vi "Motors 1.vi"(2 "Motors Visa Ref":refnum<visa-resource-name>="COM7") -> ()   [LabVIEW 2010]
panel:
  out "output cluster":T1
  in  "Cluster":T2
  in  "Y Speed (mm/s)":dbl=1.0 min=0.0
  in  "Delta Y (mm)":dbl=1.0
  in  "Theta Speed (deg/s)":dbl=1.0 min=0.0
  in  "Delta Theta (deg)":dbl=1.0
  in  "(mm/s)":dbl min=0.4
  in  "(mm/s) 3":dbl min=0.4
  in  "(mm/s) 2":dbl min=4.0
  in  "(degrees/s)":dbl min=8.0
  in  "X Set Slew Speed":bool
  in  "Y Set Slew Speed":bool
  in  "Z Set Slew Speed":bool
  in  "Theta Set Slew Speed":bool
  in  "Go To Saved Position":bool
  in  "Defined Positions":i32(listbox)
  in  "Steps to deactivate hard limit after finding datums":dbl=500.0
  out "Loop i":i32
types:
  T1 = cluster{"Set Jogger?":refnum<vi>, "Normal":refnum<vi>, "Fast":refnum<vi>, "Jogger Axis":refnum<vi>, "X Multiplier":refnum<vi>, "Y Multiplier":refnum<vi>, "Z Multiplier":refnum<vi>, "Theta Multiplier":refnum<vi>, "Need to Update Motor Parameters":refnum<vi>}
  T2 = cluster{"Stop X?":refnum<vi>, "Stop Y?":refnum<vi>, "Stop Z?":refnum<vi>, "Stop Theta?":refnum<vi>, "Backlash?":refnum<vi>, "Backlash X":refnum<vi>, "Backlash Y":refnum<vi>, "Backlash Z":refnum<vi>, "Backlash Theta":refnum<vi>, "Manual IO?":refnum<vi>, "Manual Communication is Active\n(Close Before Ending Program)":refnum<vi>, "Reset Motors?":refnum<vi>, "Set Jogger?":refnum<vi>, "Normal":refnum<vi>, "Fast":refnum<vi>, "Jogger Axis":refnum<vi>, "Redefine Origin as Current Location?":refnum<vi>, "Save Current Motor Parameters?":refnum<vi>, "Find Datums Nearest Hard Limits?":refnum<vi>, "Saved Limits":refnum<vi>, "Use Datums Nearest Hard Limits to Reset Origin?":refnum<vi>, "X Go?":refnum<vi>, "Y Go?":refnum<vi>, "Z Go?":refnum<vi>, "Theta Go?":refnum<vi>, "Jog-Mode":refnum<vi>, "x+?":refnum<vi>, "x-?":refnum<vi>, "y+?":refnum<vi>, "y-?":refnum<vi>, "z+?":refnum<vi>, "z-?":refnum<vi>, "theta+?":refnum<vi>, "theta-?":refnum<vi>, "X Set Slew Speed?":refnum<vi>, "(mm/s)":refnum<vi>, "Y Set Slew Speed?":refnum<vi>, "(mm/s)":refnum<vi>, "Z Set Slew Speed?":refnum<vi>, "(mm/s)":refnum<vi>, "Theta Set Slew Speed?":refnum<vi>, "(degrees/s)":refnum<vi>, "Go To Saved Position?":refnum<vi>, "Defined Positions":refnum<vi>, "Need to Update Motor Parameters":refnum<vi>, "X Jogger Normal Speed":refnum<vi>, "X Jogger Fast Speed":refnum<vi>, "Y Jogger Normal Speed":refnum<vi>, "Y Jogger Fast Speed":refnum<vi>, "Z Jogger Normal Speed":refnum<vi>, "Z Jogger Fast Speed":refnum<vi>, "Theta Jogger Normal Speed":refnum<vi>, "Theta Jogger Fast Speed":refnum<vi>, "X Moving":refnum<vi>, "Y Moving":refnum<vi>, "Z Moving":refnum<vi>, "Theta Moving":refnum<vi>, "X Slew Speed (mm or degree/s)":refnum<vi>, "Y Slew Speed (mm or degree/s)":refnum<vi>, "Z Slew Speed (mm or degree/s)":refnum<vi>, "Theta Slew Speed (mm or degree/s)":refnum<vi>, "X-Axis (mm)":refnum<vi>, "Y-Axis (mm)":refnum<vi>, "Z-Axis (mm)":refnum<vi>, "Theta (deg)":refnum<vi>, "X Multiplier":refnum<vi>, "Y Multiplier":refnum<vi>, "Z Multiplier":refnum<vi>, "Theta Multiplier":refnum<vi>, "Motors Online":refnum<vi>, "Motors Status":refnum<vi>, "Status X":refnum<vi>, "Status Y":refnum<vi>, "Status Z":refnum<vi>, "Status Theta":refnum<vi>, "Motors error":refnum<vi>, "QUIT":refnum<vi>, "EMERGENCY":refnum<vi>, "X Go To":refnum<vi>, "Y Go To":refnum<vi>, "Z Go To":refnum<vi>, "Theta Go To":refnum<vi>, "Delta X (mm)":refnum<vi>, "Delta Y (mm)":refnum<vi>, "Delta Z (mm)":refnum<vi>, "Delta Theta (deg)":refnum<vi>, "X Speed (mm/s)":refnum<vi>, "Y Speed (mm/s)":refnum<vi>, "Z Speed (mm/s)":refnum<vi>, "Theta Speed (deg/s)":refnum<vi>, "x+":refnum<vi>, "x-":refnum<vi>, "y+":refnum<vi>, "y-":refnum<vi>, "z+":refnum<vi>, "z-":refnum<vi>, "theta+":refnum<vi>, "theta-":refnum<vi>}
  T3 = cluster{"Stop X?":refnum<vi>, "Stop Y?":refnum<vi>, "Stop Z?":refnum<vi>, "Stop Theta?":refnum<vi>}
  T4 = cluster{"Backlash?":refnum<vi>, "Backlash X":refnum<vi>, "Backlash Y":refnum<vi>, "Backlash Z":refnum<vi>, "Backlash Theta":refnum<vi>}
  T5 = cluster{"EMERGENCY":refnum<vi>, "Manual IO?":refnum<vi>, "Manual Communication is Active\n(Close Before Ending Program)":refnum<vi>, "Reset Motors?":refnum<vi>}
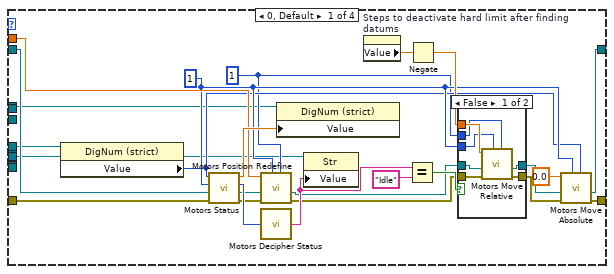
[diagram p4: hidden frame]
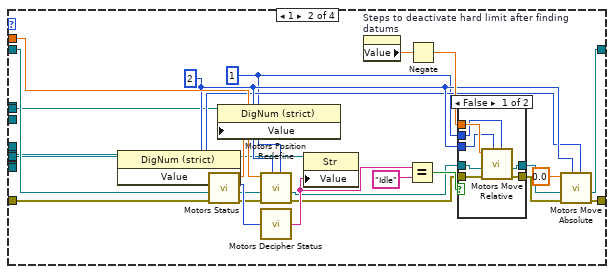
[diagram p6: hidden frame]
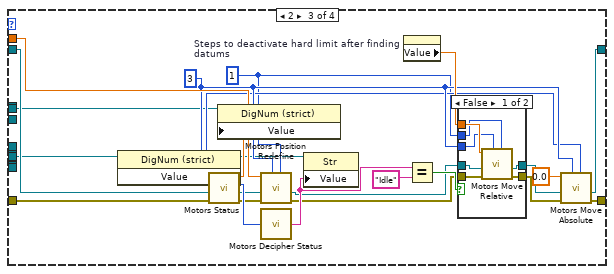
[diagram p8: hidden frame]
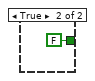
[diagram p12: hidden frame]
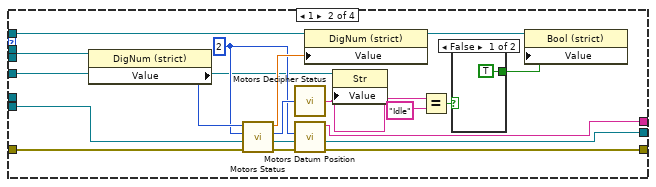
[diagram p13: hidden frame]
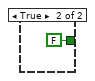
[diagram p14: hidden frame]
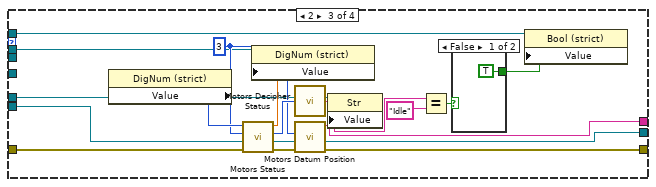
[diagram p15: hidden frame]
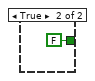
[diagram p16: hidden frame]
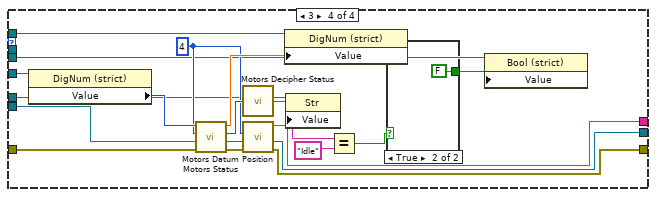
[diagram p17: hidden frame]
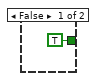
[diagram p18: hidden frame]
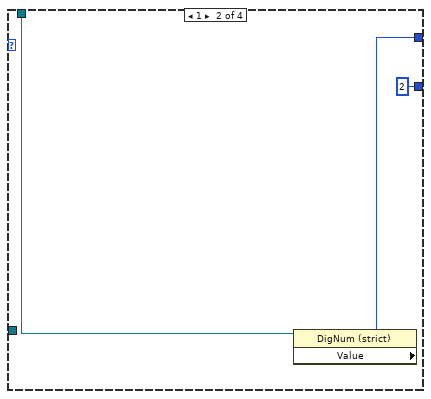
[diagram p19: hidden frame]
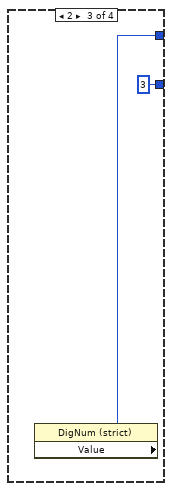
[diagram p20: hidden frame]
diagram:
  n1 = Unbundle("Cluster") -> ("Stop X?"=w27:refnum<vi>, "Stop Y?"=w26:refnum<vi>, "Stop Z?"=w25:refnum<vi>, "Stop Theta?"=w24:refnum<vi>, "Backlash?"=w23:refnum<vi>, "Backlash X"=w22:refnum<vi>, "Backlash Y"=w21:refnum<vi>, "Backlash Z"=w20:refnum<vi>, "Backlash Theta"=w19:refnum<vi>, "Manual IO?"=w17:refnum<vi>, "Manual Communication is Active\n(Close Before Ending Program)"=w16:refnum<vi>, "Reset Motors?"=w15:refnum<vi>, "Set Jogger?"=w10:refnum<vi>, "Normal"=w9:refnum<vi>, "Fast"=w8:refnum<vi>, "Jogger Axis"=w7:refnum<vi>, "Redefine Origin as Current Location?"=w68:refnum<vi>, "Save Current Motor Parameters?"=w67:refnum<vi>, "Find Datums Nearest Hard Limits?"=w66:refnum<vi>, "Saved Limits"=w65:refnum<vi>, "Use Datums Nearest Hard Limits to Reset Origin?"=w64:refnum<vi>, "X Go?"=w55:refnum<vi>, "Y Go?"=w52:refnum<vi>, "Z Go?"=w51:refnum<vi>, "Theta Go?"=w49:refnum<vi>, "Jog-Mode"=w47:refnum<vi>, "x+?"=w40:refnum<vi>, "x-?"=w41:refnum<vi>, "y+?"=w39:refnum<vi>, "y-?"=w38:refnum<vi>, "Need to Update Motor Parameters"=w1:refnum<vi>, "X Moving"=w46:refnum<vi>, "Y Moving"=w29:refnum<vi>, "Z Moving"=w63:refnum<vi>, "Theta Moving"=w62:refnum<vi>, "X-Axis (mm)"=w43:refnum<vi>, "Y-Axis (mm)"=w36:refnum<vi>, "Z-Axis (mm)"=w61:refnum<vi>, "Theta (deg)"=w59:refnum<vi>, "X Multiplier"=w6:refnum<vi>, "Y Multiplier"=w5:refnum<vi>, "Z Multiplier"=w4:refnum<vi>, "Theta Multiplier"=w2:refnum<vi>, "Motors Online"=w69:refnum<vi>, "Motors Status"=w71:refnum<vi>, "Status X"=w42:refnum<vi>, "Status Y"=w30:refnum<vi>, "Status Z"=w60:refnum<vi>, "Status Theta"=w58:refnum<vi>, "Motors error"=w13:refnum<vi>, "QUIT"=w73:refnum<vi>, "EMERGENCY"=w14:refnum<vi>, "X Go To"=w54:refnum<vi>, "Y Go To"=w53:refnum<vi>, "Z Go To"=w50:refnum<vi>, "Theta Go To"=w48:refnum<vi>, "Delta X (mm)"=w45:refnum<vi>, "Delta Y (mm)"=w28:refnum<vi>, "X Speed (mm/s)"=w44:refnum<vi>, "Y Speed (mm/s)"=w37:refnum<vi>, "x+"=w34:refnum<vi>, "x-"=w33:refnum<vi>, "y+"=w32:refnum<vi>, "y-"=w31:refnum<vi>)  [unwired: 34 out]
  n2 = property on="Property Node" class="Bool (strict)"(reference=w1, "Value"=TRUE) -> (reference out=w57:refnum<vi>)  [unwired: 1 in, 1 out]
  n3 = Bundle("Stop X?"=w27, "Stop Y?"=w26, "Stop Z?"=w25, "Stop Theta?"=w24) -> (w12:T3)  [unwired: 1 in]
  n4 = Bundle("Backlash?"=w23, "Backlash X"=w22, "Backlash Y"=w21, "Backlash Z"=w20, "Backlash Theta"=w19) -> (w18:T4)  [unwired: 1 in]
  n5 = Bundle("EMERGENCY"=w14, "Manual IO?"=w17, "Manual Communication is Active\n(Close Before Ending Program)"=w16, "Reset Motors?"=w15) -> (w11:T5)  [unwired: 1 in]
  n6 = Bundle("Set Jogger?"=w10, "Normal"=w9, "Fast"=w8, "Jogger Axis"=w7, "X Multiplier"=w6, "Y Multiplier"=w5, "Z Multiplier"=w4, "Theta Multiplier"=w2, "Need to Update Motor Parameters"=w1) -> (w3:T1)  [unwired: 1 in]
  "output cluster" <- w3
  n7 = call "Motors Open.vi"("VISA in"="Motors Visa Ref") -> ("error out"=w77:errorcluster, "VISA out"=w74:refnum<visa-resource-name>)  [unwired: 1 in]
  n8 = call <vilib>:"Simple Error Handler.vi"("error in (no error)"=w77) -> ("error?"=w76:bool, "error out"=w78:errorcluster)  [unwired: 4 in, 3 out]
  n9 = property on="Property Node" class="Str"(reference=w71, "Value"="Opening Communications") -> (reference out=w72:refnum<vi>)  [unwired: 1 in, 1 out]
  n10 = property on="Property Node" class="Clust (strict)"(reference=w13, "Value"=w78) -> ()  [unwired: 1 in, 2 out]
  n11 = Not(x=w76) -> (.not. x?=w75:bool)
  n12 = case shown="True" w75 {
    tunnel: w72 -> [_ w153]
    tunnel: w74 -> [_ w152]
    tunnel: w13 -> [_ w151]
    tunnel: w73 -> [_ w150]
    tunnel: w14 -> [_ w149]
    tunnel: w6 -> [_ w148]
    tunnel: w5 -> [_ w147]
    tunnel: w2 -> [_ w146]
    tunnel: w57 -> [_ w145]
    tunnel: w68 -> [_ w144]
    tunnel: w67 -> [_ w143]
    tunnel: w66 -> [_ w142]
    tunnel: w6 -> [_ w140]
    tunnel: w43 -> [_ w139]
    tunnel: w42 -> [_ w138]
    tunnel: w46 -> [_ w137]
    tunnel: w65 -> [_ w136]
    tunnel: w64 -> [_ w135]
    tunnel: w29 -> [_ w134]
    tunnel: w63 -> [_ w133]
    tunnel: w62 -> [_ w132]
    tunnel: w6 -> [_ w131]
    tunnel: w5 -> [_ w130]
    tunnel: w2 -> [_ w129]
    tunnel: w43 -> [_ w128]
    tunnel: w36 -> [_ w127]
    tunnel: w61 -> [_ w126]
    tunnel: w42 -> [_ w125]
    tunnel: w30 -> [_ w124]
    tunnel: w60 -> [_ w123]
    tunnel: w59 -> [_ w122]
    tunnel: w58 -> [_ w121]
    tunnel: w55 -> [_ w120]
    tunnel: w6 -> [_ w119]
    tunnel: w54 -> [_ w118]
    tunnel: w5 -> [_ w117]
    tunnel: w53 -> [_ w116]
    tunnel: w52 -> [_ w115]
    tunnel: w51 -> [_ w114]
    tunnel: w50 -> [_ w113]
    tunnel: w49 -> [_ w112]
    tunnel: w2 -> [_ w111]
    tunnel: w48 -> [_ w110]
    tunnel: w41 -> [_ w109]
    tunnel: w47 -> [_ w108]
    tunnel: w46 -> [_ w107]
    tunnel: w45 -> [_ w106]
    tunnel: w6 -> [_ w105]
    tunnel: w44 -> [_ w104]
    tunnel: w43 -> [_ w103]
    tunnel: w40 -> [_ w102]
    tunnel: w41 -> [_ w101]
    tunnel: w42 -> [_ w100]
    tunnel: w41 -> [_ w99]
    tunnel: w40 -> [_ w98]
    tunnel: w40 -> [_ w97]
    tunnel: w39 -> [_ w96]
    tunnel: w38 -> [_ w95]
    tunnel: w5 -> [_ w94]
    tunnel: w37 -> [_ w93]
    tunnel: w36 -> [_ w92]
    tunnel: w34 -> [_ w91]
    tunnel: w33 -> [_ w90]
    tunnel: w32 -> [_ w89]
    tunnel: w31 -> [_ w88]
    tunnel: w30 -> [_ w87]
    tunnel: w29 -> [_ w86]
    tunnel: w28 -> [_ w85]
    tunnel: w5 -> [_ w84]
    tunnel: w18 -> [_ w83]
    tunnel: w12 -> [_ w82]
    tunnel: w11 -> [_ w81]
    tunnel: w3 -> [_ w80]
    frame False {
    }
    frame True {
      n13 = property on="Property Node" class="Str"(reference=w153, "Value"="Running") -> (reference out=w141:refnum<vi>)  [unwired: 1 in, 1 out]
      n14 = while {
        shift-right: _ -> [_]
        shift-left: w152 -> [w166]
        tunnel: w151 -> [w321]
        tunnel: w150 -> [w259]
        tunnel: w149 -> [_]
        tunnel: w148 -> [w256]
        tunnel: w147 -> [w255]
        tunnel: w146 -> [w254]
        tunnel: w145 -> [w253]
        tunnel: w144 -> [w251]
        tunnel: w143 -> [w250]
        tunnel: w142 -> [w248]
        tunnel: w141 -> [w247]
        tunnel: w140 -> [w246]
        tunnel: w139 -> [w245]
        tunnel: w138 -> [w244]
        tunnel: w137 -> [w243]
        tunnel: w136 -> [w242]
        tunnel: w135 -> [w222]
        tunnel: w134 -> [w240]
        tunnel: w133 -> [w239]
        tunnel: w132 -> [w238]
        tunnel: w131 -> [w235]
        tunnel: w130 -> [w234]
        tunnel: w129 -> [w233]
        tunnel: w128 -> [w232]
        tunnel: w127 -> [w231]
        tunnel: w126 -> [w230]
        tunnel: w125 -> [w229]
        tunnel: w124 -> [w228]
        tunnel: w123 -> [w227]
        tunnel: w122 -> [w226]
        tunnel: w121 -> [w225]
        tunnel: w120 -> [w223]
        tunnel: w119 -> [w214]
        tunnel: w118 -> [w213]
        tunnel: w117 -> [w212]
        tunnel: w116 -> [w211]
        tunnel: w115 -> [w209]
        tunnel: w114 -> [w206]
        tunnel: w113 -> [w204]
        tunnel: w112 -> [w202]
        tunnel: w111 -> [w198]
        tunnel: w110 -> [w200]
        tunnel: w109 -> [w199]
        tunnel: w108 -> [w196]
        tunnel: w107 -> [w195]
        tunnel: w106 -> [w194]
        tunnel: w105 -> [w193]
        tunnel: w104 -> [w192]
        tunnel: w103 -> [w191]
        tunnel: w102 -> [w190]
        tunnel: w101 -> [w189]
        tunnel: w100 -> [w188]
        tunnel: w99 -> [w187]
        tunnel: w98 -> [w186]
        tunnel: w97 -> [w185]
        tunnel: w96 -> [w184]
        tunnel: w95 -> [w183]
        tunnel: w94 -> [w182]
        tunnel: w93 -> [w181]
        tunnel: w92 -> [w180]
        tunnel: w91 -> [w176]
        tunnel: w90 -> [w175]
        tunnel: w89 -> [w174]
        tunnel: w88 -> [w173]
        tunnel: w87 -> [w172]
        tunnel: w86 -> [w169]
        tunnel: w85 -> [w168]
        tunnel: w84 -> [w167]
        tunnel: w83 -> [w162]
        tunnel: w82 -> [w164]
        tunnel: w81 -> [w160]
        tunnel: w80 -> [w155]
        i -> [w260]
        stop <- w322 stop-if-true
        # "This loop contains all of the code that has to communicate directly with the manipulator motor controllers.  They are arranged linearly to ensure multiple serial I/O's are never attempted simultaneously.  Note that this loop executes very slowly (each serial I/O takes about 1/20 sec)."
        n15 = property on="Property Node" class="Bool (strict)"(reference=w184) -> (reference out=w170:refnum<vi>, "Value"=w272:bool)  [unwired: 1 in, 1 out]
        n16 = property on="Property Node" class="Bool (strict)"(reference=w183) -> (reference out=w171:refnum<vi>, "Value"=w273:bool)  [unwired: 1 in, 1 out]
        n17 = property on="Property Node" class="Clust (strict)"(reference=w321) -> ("Value"=w163:errorcluster)  [unwired: 1 in, 2 out]
        n18 = Or(x=w272, y=w273) -> (x .or. y?=w303:bool)
        n19 = property on="Property Node" class="Bool (strict)"(reference=w199) -> (reference out=w178:refnum<vi>, "Value"=w276:bool)  [unwired: 1 in, 1 out]
        n20 = property on="Property Node" class="Bool (strict)"(reference=w186) -> (reference out=w177:refnum<vi>, "Value"=w277:bool)  [unwired: 1 in, 1 out]
        n21 = call "Motors Sub 01.vi"("Cluster"=w164, "Error In"=w163, "VISA in"=w166) -> ("error out"=w161:errorcluster, "VISA out"=w165:refnum<visa-resource-name>)  [unwired: 7 in]
        n22 = property on="Property Node" class="Bool (strict)"(reference=w196) -> ("Value"=w197:bool)  [unwired: 1 in, 2 out]
        n23 = call "Motors Sub 02.vi"("Cluster"=w162, "error in"=w161, "VISA in"=w165) -> ("error out"=w158:errorcluster, "VISA out"=w159:refnum<visa-resource-name>)  [unwired: 7 in]
        n24 = property on="Property Node" class="Bool (strict)"(reference=w223) -> (reference out=w179:refnum<vi>, "Value"=w224:bool)  [unwired: 1 in, 1 out]
        n25 = property on="Property Node" class="Bool (strict)"(reference=w259) -> ("Value"=w322:bool)  [unwired: 1 in, 2 out]
        n26 = Or(x=w277, y=w276) -> (x .or. y?=w309:bool)
        n27 = call "Motors Sub 03.vi"("Cluster"=w160, "error in"=w158, "VISA in"=w159) -> ("error out"=w156:errorcluster, "VISA out"=w157:refnum<visa-resource-name>)  [unwired: 7 in]
        n28 = property on="Property Node" class="DigNum (strict)" props=["Value"]() -> ()  [unwired: 2 in, 3 out]
        n29 = call "Motors Sub 04.vi"("Cluster"=w155, "error in"=w156, "VISA in"=w157) -> ()  [unwired: 7 in, 2 out]
        n30 = property on="Property Node" class="Bool (strict)"(reference=w209) -> (reference out=w208:refnum<vi>, "Value"=w210:bool)  [unwired: 1 in, 1 out]
        n31 = property on="Property Node" class="Bool (strict)"(reference=w206) -> (reference out=w205:refnum<vi>, "Value"=w207:bool)  [unwired: 1 in, 1 out]
        n32 = property on="Property Node" class="Bool (strict)"(reference=w202) -> (reference out=w201:refnum<vi>, "Value"=w203:bool)  [unwired: 1 in, 1 out]
        n33 = property on="Property Node" class="Ring (strict)"() -> ("Value"=w257:u16)  [unwired: 2 in, 2 out]
        n34 = property on="Property Node" class="Bool (strict)"() -> ("Value"=w274:bool)  [unwired: 2 in, 2 out]
        n35 = property on="Property Node" class="Bool (strict)"() -> ("Value"=w275:bool)  [unwired: 2 in, 2 out]
        n36 = case shown="0, Default" w257 {
          tunnel: [u32 1 u32 2 u32 3 u32 4] -> w269
          tunnel: [w719 w722 w724 w727] -> w268
          tunnel: w256 -> [w718 _ _ _]
          tunnel: w255 -> [_ w721 _ _]
          tunnel: w254 -> [_ _ _ w726]
          frame 0, Default {
            n37 = property on="Property Node" class="DigNum (strict)"(reference=w718) -> ("Value"=w719:u32)  [unwired: 1 in, 2 out]
          }
          frame 1 {
            n38 = property on="Property Node" class="DigNum (strict)"(reference=w721) -> ("Value"=w722:u32)  [unwired: 1 in, 2 out]
          }
          frame 2 {
            n39 = property on="Property Node" class="DigNum (strict)"() -> ("Value"=w724:u32)  [unwired: 2 in, 2 out]
          }
          frame 3 {
            n40 = property on="Property Node" class="DigNum (strict)"(reference=w726) -> ("Value"=w727:u32)  [unwired: 1 in, 2 out]
          }
        }
        n41 = Or(x=w275, y=w274) -> (x .or. y?=w306:bool)
        n42 = property on="Property Node" class="Bool (strict)"() -> (reference out=w215:refnum<vi>, "Value"=w258:bool)  [unwired: 2 in, 1 out]
        n43 = case shown="True" w258 {
          tunnel: [_ w1371] -> w319
          tunnel: [_ w1368] -> w320
          tunnel: w269 -> [_ w1370]
          tunnel: w268 -> [_ w1369]
          tunnel: w253 -> [_ w1366]
          tunnel: w215 -> [_ w1362]
          frame False {
          }
          frame True {
            n44 = property on="Property Node" class="DigNum (strict)"() -> ("Value"=w1365:dbl)  [unwired: 2 in, 2 out]
            n45 = property on="Property Node" class="DigNum (strict)"() -> ("Value"=w1364:dbl)  [unwired: 2 in, 2 out]
            n46 = property on="Property Node" class="Bool (strict)"(reference=w1366, "Value"=TRUE ("Need to Update Motor Parameters")) -> ()  [unwired: 1 in, 2 out]
            n47 = call "Motors Jogger Speed.vi"("Axis Multiplier"=w1369, "Axis"=w1370, "Fast Speed (mm or degree/sec)"=w1364, "Normal Speed (mm or degree/sec)"=w1365) -> ("error out"=w1371:errorcluster, "VISA out"=w1368:refnum<visa-resource-name>)  [unwired: 6 in]
            n48 = property on="Property Node" class="Bool (strict)"(reference=w1362, "Value"=FALSE) -> ()  [unwired: 1 in, 2 out]
          }
        }
        n49 = property on="Property Node" class="Bool (strict)"(reference=w251) -> (reference out=w216:refnum<vi>, "Value"=w252:bool)  [unwired: 1 in, 1 out]
        n50 = property on="Property Node" class="Bool (strict)"(reference=w250) -> (reference out=w218:refnum<vi>, "Value"=w217:bool)  [unwired: 1 in, 1 out]
        n51 = case shown="True" w252 {
          tunnel: w320 -> [w1354 w1361]
          tunnel: w319 -> [w1355 w1357]
          tunnel: [w1355 w1359] -> w219
          tunnel: [w1354 w1360] -> w318
          tunnel: w216 -> [_ w1356]
          frame False {
          }
          frame True {
            n52 = property on="Property Node" class="Bool (strict)"(reference=w1356, "Value"=FALSE) -> ()  [unwired: 1 in, 2 out]
            n53 = call "Motors Redefine Origin.vi"("error in"=w1357, "VISA in"=w1361) -> ("error out"=w1359:errorcluster, "VISA out"=w1360:refnum<visa-resource-name>)
          }
        }
        n54 = property on="Property Node" class="Bool (strict)"(reference=w248) -> (reference out=w221:refnum<vi>, "Value"=w249:bool)  [unwired: 1 in, 1 out]
        n55 = case shown="True" w217 {
          tunnel: w219 -> [w1347 w1353]
          tunnel: [w1347 w1352] -> w266
          tunnel: w318 -> [w1346 w1351]
          tunnel: [w1346 w1350] -> w265
          tunnel: w218 -> [_ w1349]
          frame False {
          }
          frame True {
            n56 = property on="Property Node" class="Bool (strict)"(reference=w1349, "Value"=FALSE) -> ()  [unwired: 1 in, 2 out]
            n57 = call "Motors Save.vi"("error in"=w1353, "VISA in"=w1351) -> ("error out"=w1352:errorcluster, "VISA out"=w1350:refnum<visa-resource-name>)
          }
        }
        n58 = case shown="True" w249 {
          tunnel: w266 -> [w536 w566]
          tunnel: [w536 w564] -> w263
          tunnel: [w535 w565] -> w261
          tunnel: w265 -> [w535 w567]
          tunnel: w247 -> [w533 w559]
          tunnel: w246 -> [_ w556]
          tunnel: w245 -> [_ w555]
          tunnel: w244 -> [_ w554]
          tunnel: w243 -> [_ w553]
          tunnel: w242 -> [w534 w552]
          tunnel: w234 -> [_ w551]
          tunnel: w231 -> [_ w550]
          tunnel: w228 -> [_ w549]
          tunnel: w240 -> [_ w548]
          tunnel: w230 -> [_ w547]
          tunnel: w227 -> [_ w546]
          tunnel: w239 -> [_ w545]
          tunnel: w233 -> [_ w544]
          tunnel: w226 -> [_ w543]
          tunnel: w225 -> [_ w542]
          tunnel: w238 -> [_ w541]
          tunnel: [w534 w540] -> w237
          tunnel: [w533 w539] -> w236
          tunnel: w221 -> [_ w538]
          frame False {
          }
          frame True {
            n59 = flat-sequence {
              tunnel: w566 -> [w572]
              tunnel: w567 -> [w573]
              tunnel: [w573] -> w563
              tunnel: [w572] -> w562
              tunnel: w559 -> [w569]
              tunnel: [w568] -> w557
              tunnel: w563 -> [w608]
              tunnel: w562 -> [w607]
              tunnel: [w603] -> w561
              tunnel: [w602] -> w560
              tunnel: [w592] -> w558
              tunnel: w557 -> [w592]
              tunnel: w556 -> [w591]
              tunnel: w555 -> [w590]
              tunnel: w554 -> [w589]
              tunnel: w553 -> [w588]
              tunnel: w552 -> [w586]
              tunnel: w551 -> [w585]
              tunnel: w550 -> [w584]
              tunnel: w549 -> [w583]
              tunnel: w548 -> [w582]
              tunnel: w547 -> [w581]
              tunnel: w546 -> [w580]
              tunnel: w545 -> [w579]
              tunnel: w544 -> [w578]
              tunnel: w543 -> [w577]
              tunnel: w542 -> [w576]
              tunnel: w541 -> [w575]
              tunnel: [w574] -> w540
              tunnel: [w716] -> w564
              tunnel: [w717] -> w565
              tunnel: w561 -> [w717]
              tunnel: w560 -> [w716]
              tunnel: w558 -> [w714]
              tunnel: [w713] -> w539
              frame #0 {
                n60 = call <vilib>:"Set Busy.vi"("disable click? (T)"=FALSE) -> ()  [unwired: 9 in, 2 out]
                n61 = property on="Property Node" class="Str"(reference=w569, "Value"="Finding Datums Nearest Hard Limits\nThis May Take a Few Minutes" ("Status")) -> (reference out=w568:refnum<vi>)  [unwired: 1 in, 1 out]
              }
              frame #1 {
                n62 = call "Motors Find Datums.vi"("error in"=w607, "VISA in"=w608) -> ("error out"=w604:errorcluster, "VISA out"=w605:refnum<visa-resource-name>)
                n63 = for {
                  N: 4 -> [_]
                  shift-right: [w627] -> w602
                  shift-left: w604 -> [w628]
                  shift-right: [w626] -> w603
                  shift-left: w605 -> [w629]
                  tunnel: [w625] -> w594 mode=indexing
                  tunnel: w591 -> [w623]
                  tunnel: w590 -> [w622]
                  tunnel: w589 -> [w621]
                  tunnel: w588 -> [w620]
                  tunnel: w585 -> [w619]
                  tunnel: w584 -> [w618]
                  tunnel: w583 -> [w617]
                  tunnel: w582 -> [w616]
                  tunnel: w581 -> [w615]
                  tunnel: w580 -> [w614]
                  tunnel: w579 -> [w613]
                  tunnel: w578 -> [w612]
                  tunnel: w577 -> [w611]
                  tunnel: w576 -> [w610]
                  tunnel: w575 -> [w609]
                  i -> [w624]
                  n64 = case shown="0, Default" w624 {
                    tunnel: w628 -> [w642 w663 w683 w704]
                    tunnel: w629 -> [w643 w664 w684 w705]
                    tunnel: [w636 w657 w676 w697] -> w627
                    tunnel: [w637 w658 w677 w698] -> w626
                    tunnel: [w634 w655 w680 w701] -> w625
                    tunnel: w623 -> [w633 _ _ _]
                    tunnel: w622 -> [w632 _ _ _]
                    tunnel: w621 -> [w631 _ _ _]
                    tunnel: w620 -> [w630 _ _ _]
                    tunnel: w619 -> [_ w654 _ _]
                    tunnel: w618 -> [_ w653 _ _]
                    tunnel: w617 -> [_ w652 _ _]
                    tunnel: w616 -> [_ w651 _ _]
                    tunnel: w615 -> [_ _ w674 _]
                    tunnel: w614 -> [_ _ w673 _]
                    tunnel: w613 -> [_ _ w672 _]
                    tunnel: w612 -> [_ _ _ w695]
                    tunnel: w611 -> [_ _ _ w694]
                    tunnel: w610 -> [_ _ _ w693]
                    tunnel: w609 -> [_ _ _ w692]
                    frame 0, Default {
                      w635 = 1 ("Axis")
                      n65 = property on="Property Node" class="DigNum (strict)"(reference=w633) -> ("Value"=w641:u32)  [unwired: 1 in, 2 out]
                      n66 = call "Motors Status.vi"("error in"=w642, "VISA in"=w643, "Axis"=w635, "Axis Multiplier"=w641) -> ("error out"=w638:errorcluster, "VISA out"=w639:refnum<visa-resource-name>, "OS"=w648:i32, "Actual Position (mm or deg)"=w640:dbl)  [unwired: 3 in]
                      n67 = property on="Property Node" class="DigNum (strict)"(reference=w632, "Value"=w640) -> ()  [unwired: 1 in, 2 out]
                      n68 = call "Motors Decipher Status.vi"("OS"=w648) -> ("Status"=w647:string)
                      n69 = call "Motors Datum Position.vi"("error in"=w638, "VISA in"=w639, "Axis"=w635) -> ("error out"=w636:errorcluster, "VISA out"=w637:refnum<visa-resource-name>, "Datum Position (steps)"=w634:string)  [unwired: 5 in]
                      n70 = property on="Property Node" class="Str"(reference=w631, "Value"=w647) -> ()  [unwired: 1 in, 2 out]
                      n71 = Equal?(x=w647, y="Idle") -> (x = y?=w645:bool)
                      n72 = case shown="False" w645 {
                        tunnel: [TRUE FALSE] -> w644
                        frame False {
                        }
                        frame True {
                        }
                      }
                      n73 = property on="Property Node" class="Bool (strict)"(reference=w630, "Value"=w644) -> ()  [unwired: 1 in, 2 out]
                    }
                    frame 1 {
                      w656 = 2 ("Axis")
                      n74 = property on="Property Node" class="DigNum (strict)"(reference=w654) -> ("Value"=w662:u32)  [unwired: 1 in, 2 out]
                      n75 = call "Motors Status.vi"("error in"=w663, "VISA in"=w664, "Axis"=w656, "Axis Multiplier"=w662) -> ("error out"=w659:errorcluster, "VISA out"=w660:refnum<visa-resource-name>, "OS"=w669:i32, "Actual Position (mm or deg)"=w661:dbl)  [unwired: 3 in]
                      n76 = call "Motors Decipher Status.vi"("OS"=w669) -> ("Status"=w667:string)
                      n77 = call "Motors Datum Position.vi"("error in"=w659, "VISA in"=w660, "Axis"=w656) -> ("error out"=w657:errorcluster, "VISA out"=w658:refnum<visa-resource-name>, "Datum Position (steps)"=w655:string)  [unwired: 5 in]
                      n78 = property on="Property Node" class="DigNum (strict)"(reference=w653, "Value"=w661) -> ()  [unwired: 1 in, 2 out]
                      n79 = property on="Property Node" class="Str"(reference=w652, "Value"=w667) -> ()  [unwired: 1 in, 2 out]
                      n80 = Equal?(x=w667, y="Idle") -> (x = y?=w666:bool)
                      n81 = case shown="False" w666 {
                        tunnel: [TRUE FALSE] -> w665
                        frame False {
                        }
                        frame True {
                        }
                      }
                      n82 = property on="Property Node" class="Bool (strict)"(reference=w651, "Value"=w665) -> ()  [unwired: 1 in, 2 out]
                    }
                    frame 2 {
                      w675 = 3 ("Axis")
                      n83 = property on="Property Node" class="DigNum (strict)"() -> ("Value"=w682:u32)  [unwired: 2 in, 2 out]
                      n84 = call "Motors Status.vi"("error in"=w683, "VISA in"=w684, "Axis"=w675, "Axis Multiplier"=w682) -> ("error out"=w678:errorcluster, "VISA out"=w679:refnum<visa-resource-name>, "OS"=w689:i32, "Actual Position (mm or deg)"=w681:dbl)  [unwired: 3 in]
                      n85 = property on="Property Node" class="DigNum (strict)"(reference=w674, "Value"=w681) -> ()  [unwired: 1 in, 2 out]
                      n86 = call "Motors Decipher Status.vi"("OS"=w689) -> ("Status"=w687:string)
                      n87 = call "Motors Datum Position.vi"("error in"=w678, "VISA in"=w679, "Axis"=w675) -> ("error out"=w676:errorcluster, "VISA out"=w677:refnum<visa-resource-name>, "Datum Position (steps)"=w680:string)  [unwired: 5 in]
                      n88 = property on="Property Node" class="Str"(reference=w673, "Value"=w687) -> ()  [unwired: 1 in, 2 out]
                      n89 = Equal?(x=w687, y="Idle") -> (x = y?=w686:bool)
                      n90 = case shown="False" w686 {
                        tunnel: [TRUE FALSE] -> w685
                        frame False {
                        }
                        frame True {
                        }
                      }
                      n91 = property on="Property Node" class="Bool (strict)"(reference=w672, "Value"=w685) -> ()  [unwired: 1 in, 2 out]
                    }
                    frame 3 {
                      w696 = 4 ("Axis")
                      n92 = property on="Property Node" class="DigNum (strict)"(reference=w695) -> ("Value"=w703:u32)  [unwired: 1 in, 2 out]
                      n93 = call "Motors Status.vi"("error in"=w704, "VISA in"=w705, "Axis"=w696, "Axis Multiplier"=w703) -> ("error out"=w699:errorcluster, "VISA out"=w700:refnum<visa-resource-name>, "OS"=w710:i32, "Actual Position (mm or deg)"=w702:dbl)  [unwired: 3 in]
                      n94 = call "Motors Decipher Status.vi"("OS"=w710) -> ("Status"=w708:string)
                      n95 = call "Motors Datum Position.vi"("error in"=w699, "VISA in"=w700, "Axis"=w696) -> ("error out"=w697:errorcluster, "VISA out"=w698:refnum<visa-resource-name>, "Datum Position (steps)"=w701:string)  [unwired: 5 in]
                      n96 = property on="Property Node" class="DigNum (strict)"(reference=w694, "Value"=w702) -> ()  [unwired: 1 in, 2 out]
                      n97 = property on="Property Node" class="Str"(reference=w693, "Value"=w708) -> ()  [unwired: 1 in, 2 out]
                      n98 = Equal?(x=w708, y="Idle") -> (x = y?=w707:bool)
                      n99 = case shown="True" w707 {
                        tunnel: [TRUE FALSE] -> w706
                        frame False {
                        }
                        frame True {
                        }
                      }
                      n100 = property on="Property Node" class="Bool (strict)"(reference=w692, "Value"=w706) -> ()  [unwired: 1 in, 2 out]
                    }
                  }
                }
                n101 = Build Array (concatenate)("Limits", w594) -> (w593:string[])
                n102 = Initialize Array("", 0 ("dimension size"), 0 ("dimension size")) -> (w600:string[][])
                n103 = Build Array (concatenate)(w593, w600) -> (w598:string[][])
                n104 = property on="Property Node" class="Path"(reference=w586) -> (reference out=w574:refnum<vi>, "Value"=w587:path)  [unwired: 1 in, 1 out]
                n105 = Transpose 2D Array(2D array=w598) -> (transposed array=w597:string[][])
                n106 = call "Motors Position Rewrite.vi"("file path"=w587, "Array of Positions"=w597) -> ()  [unwired: 9 in]
              }
              frame #2 {
                n107 = call <vilib>:"Unset Busy.vi"() -> ()  [unwired: 11 in, 1 out]
                n108 = property on="Property Node" class="Str"(reference=w714, "Value"="Running" ("Status")) -> (reference out=w713:refnum<vi>)  [unwired: 1 in, 1 out]
              }
            }
            n109 = property on="Property Node" class="Bool (strict)"(reference=w538, "Value"=FALSE) -> ()  [unwired: 1 in, 2 out]
          }
        }
        n110 = property on="Property Node" class="Bool (strict)"(reference=w222) -> (reference out=w220:refnum<vi>, "Value"=w241:bool)  [unwired: 1 in, 1 out]
        n111 = case shown="True" w241 {
          tunnel: [w325 w345] -> w264
          tunnel: w263 -> [w325 w347]
          tunnel: [w324 w344] -> w262
          tunnel: w261 -> [w324 w348]
          tunnel: w237 -> [_ w343]
          tunnel: w236 -> [w323 w328]
          tunnel: w235 -> [_ w342]
          tunnel: w234 -> [_ w341]
          tunnel: w233 -> [_ w340]
          tunnel: w232 -> [_ w339]
          tunnel: w231 -> [_ w338]
          tunnel: w230 -> [_ w337]
          tunnel: w229 -> [_ w336]
          tunnel: w228 -> [_ w335]
          tunnel: w227 -> [_ w334]
          tunnel: w226 -> [_ w333]
          tunnel: w225 -> [_ w332]
          tunnel: [w323 w329] -> _
          tunnel: w220 -> [_ w327]
          frame False {
          }
          frame True {
            n112 = property on="Property Node" class="Bool (strict)"(reference=w327, "Value"=FALSE) -> ()  [unwired: 1 in, 2 out]
            n113 = flat-sequence {
              tunnel: w347 -> [w352]
              tunnel: [w352] -> w346
              tunnel: w328 -> [w350]
              tunnel: [w349] -> w330
              tunnel: w348 -> [w375]
              tunnel: w346 -> [w376]
              tunnel: [w371] -> w345
              tunnel: [w370] -> w344
              tunnel: w343 -> [w366]
              tunnel: w342 -> [w364]
              tunnel: w341 -> [w363]
              tunnel: w340 -> [w362]
              tunnel: w339 -> [w361]
              tunnel: w338 -> [w360]
              tunnel: w337 -> [w359]
              tunnel: w336 -> [w358]
              tunnel: w335 -> [w357]
              tunnel: w334 -> [w356]
              tunnel: w333 -> [w355]
              tunnel: w332 -> [w354]
              tunnel: [w353] -> w331
              tunnel: w330 -> [w353]
              tunnel: w331 -> [w531]
              tunnel: [w530] -> w329
              frame #0 {
                n114 = call <vilib>:"Set Busy.vi"() -> ()  [unwired: 10 in, 2 out]
                n115 = property on="Property Node" class="Str"(reference=w350, "Value"="Finding Datums Nearest Hard Limits\nThis May Take a Few Minutes" ("Status")) -> (reference out=w349:refnum<vi>)  [unwired: 1 in, 1 out]
              }
              frame #1 {
                n116 = property on="Property Node" class="Path"(reference=w366) -> ("Value"=w365:path)  [unwired: 1 in, 2 out]
                n117 = call "Motors Find Datums.vi"("error in"=w376, "VISA in"=w375) -> ("error out"=w373:errorcluster, "VISA out"=w374:refnum<visa-resource-name>)
                n118 = call "Motors Position Load.vi"("error in"=w373, "file path"=w365) -> ("error out"=w372:errorcluster, "Positions"=w369:string[][])
                n119 = Delete From Array(array=w369, index (row)=0) -> (array with subset deleted=w367:string[][])  [unwired: 2 in, 1 out]
                n120 = for {
                  shift-right: [w394] -> w371
                  shift-left: w372 -> [w395]
                  shift-right: [w393] -> w370
                  shift-left: w374 -> [w396]
                  tunnel: w367 -> [w392] mode=indexing
                  tunnel: w364 -> [w387]
                  tunnel: w363 -> [w386]
                  tunnel: w362 -> [w385]
                  tunnel: w361 -> [w384]
                  tunnel: w360 -> [w383]
                  tunnel: w359 -> [w382]
                  tunnel: w358 -> [w381]
                  tunnel: w357 -> [w380]
                  tunnel: w356 -> [w379]
                  tunnel: w355 -> [w378]
                  tunnel: w354 -> [w377]
                  i -> [w389]
                  n121 = Index Array(array=w392, index=0) -> (element=w391:string)
                  n122 = Fract/Exp String To Number(string=w391) -> (number=w390:dbl)  [unwired: 3 in, 1 out]
                  n123 = case shown="3" w389 {
                    tunnel: w395 -> [w416 w450 w479 w515]
                    tunnel: w396 -> [w417 w451 w480 w516]
                    tunnel: [w410 w443 w471 w508] -> w394
                    tunnel: [w411 w444 w472 w509] -> w393
                    tunnel: w390 -> [w412 w446 w482 w511]
                    tunnel: w387 -> [w399 _ _ _]
                    tunnel: w386 -> [_ w433 _ _]
                    tunnel: w385 -> [_ _ _ w499]
                    tunnel: w384 -> [w398 _ _ _]
                    tunnel: w383 -> [_ w432 _ _]
                    tunnel: w382 -> [_ _ w466 _]
                    tunnel: w381 -> [w397 _ _ _]
                    tunnel: w380 -> [_ w431 _ _]
                    tunnel: w379 -> [_ _ w465 _]
                    tunnel: w378 -> [_ _ _ w498]
                    tunnel: w377 -> [_ _ _ w497]
                    frame 0, Default {
                      w400 = u32 1 ("Axis Multiplier")
                      w402 = 1 ("Axis")
                      n124 = property on="Property Node" class="DigNum (strict)"(reference=w399) -> ("Value"=w401:u32)  [unwired: 1 in, 2 out]
                      n125 = call "Motors Status.vi"("error in"=w416, "VISA in"=w417, "Axis"=w402, "Axis Multiplier"=w401) -> ("error out"=w413:errorcluster, "VISA out"=w414:refnum<visa-resource-name>, "OS"=w421:i32, "Actual Position (mm or deg)"=w415:dbl)  [unwired: 3 in]
                      n126 = call "Motors Position Redefine.vi"("Axis Multiplier"=w400, "Axis"=w402, "error in"=w413, "VISA in"=w414, "Position (mm or deg)"=w412) -> ("error out"=w407:errorcluster, "VISA out"=w404:refnum<visa-resource-name>)  [unwired: 5 in]
                      n127 = call "Motors Decipher Status.vi"("OS"=w421) -> ("Status"=w420:string)
                      n128 = property on="Property Node" class="DigNum (strict)"(reference=w398, "Value"=w415) -> ()  [unwired: 1 in, 2 out]
                      n129 = property on="Property Node" class="Str"(reference=w397, "Value"=w420) -> ()  [unwired: 1 in, 2 out]
                      n130 = property on="Steps to deactivate hard limit after finding datums" class="DigNum (strict)"() -> ("Value"=w408:dbl)  [unwired: 2 in, 2 out]
                      n131 = Equal?(x=w420, y="Idle") -> (x = y?=w418:bool)
                      n132 = Negate(x=w408) -> (-x=w403:dbl)
                      n133 = case shown="False" w418 {
                        tunnel: w407 -> [w428 w430]
                        tunnel: [w427 w430] -> w406
                        tunnel: w404 -> [w426 w429]
                        tunnel: [w425 w429] -> w405
                        tunnel: w403 -> [w424 _]
                        tunnel: w402 -> [w423 _]
                        tunnel: w400 -> [w422 _]
                        frame False {
                          n134 = call "Motors Move Relative.vi"("Axis Multiplier"=w422, "Axis"=w423, "error in"=w428, "VISA in"=w426, "Distance (mm)"=w424) -> ("error out"=w427:errorcluster, "VISA out"=w425:refnum<visa-resource-name>)  [unwired: 5 in]
                        }
                        frame True {
                        }
                      }
                      n135 = call "Motors Move Absolute.vi"("Axis Multiplier"=w401, "Axis"=w402, "error in"=w406, "VISA in"=w405, "Position (mm or degree)"=0.0) -> ("error out"=w410:errorcluster, "VISA out"=w411:refnum<visa-resource-name>)  [unwired: 5 in]
                    }
                    frame 1 {
                      w434 = u32 1 ("Axis Multiplier")
                      w436 = 2 ("Axis")
                      n136 = property on="Property Node" class="DigNum (strict)"(reference=w433) -> ("Value"=w435:u32)  [unwired: 1 in, 2 out]
                      n137 = call "Motors Status.vi"("error in"=w450, "VISA in"=w451, "Axis"=w436, "Axis Multiplier"=w435) -> ("error out"=w447:errorcluster, "VISA out"=w448:refnum<visa-resource-name>, "OS"=w455:i32, "Actual Position (mm or deg)"=w449:dbl)  [unwired: 3 in]
                      n138 = property on="Property Node" class="DigNum (strict)"(reference=w432, "Value"=w449) -> ()  [unwired: 1 in, 2 out]
                      n139 = call "Motors Position Redefine.vi"("Axis Multiplier"=w434, "Axis"=w436, "error in"=w447, "VISA in"=w448, "Position (mm or deg)"=w446) -> ("error out"=w440:errorcluster, "VISA out"=w441:refnum<visa-resource-name>)  [unwired: 5 in]
                      n140 = call "Motors Decipher Status.vi"("OS"=w455) -> ("Status"=w453:string)
                      n141 = property on="Property Node" class="Str"(reference=w431, "Value"=w453) -> ()  [unwired: 1 in, 2 out]
                      n142 = property on="Steps to deactivate hard limit after finding datums" class="DigNum (strict)"() -> ("Value"=w442:dbl)  [unwired: 2 in, 2 out]
                      n143 = Equal?(x=w453, y="Idle") -> (x = y?=w452:bool)
                      n144 = Negate(x=w442) -> (-x=w437:dbl)
                      n145 = case shown="False" w452 {
                        tunnel: w441 -> [w462 w463]
                        tunnel: w440 -> [w461 w464]
                        tunnel: [w460 w463] -> w439
                        tunnel: [w459 w464] -> w438
                        tunnel: w437 -> [w458 _]
                        tunnel: w436 -> [w457 _]
                        tunnel: w434 -> [w456 _]
                        frame False {
                          n146 = call "Motors Move Relative.vi"("Axis Multiplier"=w456, "Axis"=w457, "error in"=w461, "VISA in"=w462, "Distance (mm)"=w458) -> ("error out"=w459:errorcluster, "VISA out"=w460:refnum<visa-resource-name>)  [unwired: 5 in]
                        }
                        frame True {
                        }
                      }
                      n147 = call "Motors Move Absolute.vi"("Axis Multiplier"=w435, "Axis"=w436, "error in"=w438, "VISA in"=w439, "Position (mm or degree)"=0.0) -> ("error out"=w443:errorcluster, "VISA out"=w444:refnum<visa-resource-name>)  [unwired: 5 in]
                    }
                    frame 2 {
                      w467 = u32 1 ("Axis Multiplier")
                      w469 = 3 ("Axis")
                      n148 = property on="Property Node" class="DigNum (strict)"() -> ("Value"=w468:u32)  [unwired: 2 in, 2 out]
                      n149 = call "Motors Status.vi"("error in"=w479, "VISA in"=w480, "Axis"=w469, "Axis Multiplier"=w468) -> ("error out"=w477:errorcluster, "VISA out"=w478:refnum<visa-resource-name>, "OS"=w487:i32, "Actual Position (mm or deg)"=w483:dbl)  [unwired: 3 in]
                      n150 = property on="Property Node" class="DigNum (strict)"(reference=w466, "Value"=w483) -> ()  [unwired: 1 in, 2 out]
                      n151 = call "Motors Position Redefine.vi"("Axis Multiplier"=w467, "Axis"=w469, "error in"=w477, "VISA in"=w478, "Position (mm or deg)"=w482) -> ("error out"=w475:errorcluster, "VISA out"=w476:refnum<visa-resource-name>)  [unwired: 5 in]
                      n152 = call "Motors Decipher Status.vi"("OS"=w487) -> ("Status"=w485:string)
                      n153 = property on="Property Node" class="Str"(reference=w465, "Value"=w485) -> ()  [unwired: 1 in, 2 out]
                      n154 = property on="Steps to deactivate hard limit after finding datums" class="DigNum (strict)"() -> ("Value"=w470:dbl)  [unwired: 2 in, 2 out]
                      n155 = Equal?(x=w485, y="Idle") -> (x = y?=w484:bool)
                      n156 = case shown="False" w484 {
                        tunnel: w476 -> [w494 w495]
                        tunnel: w475 -> [w493 w496]
                        tunnel: [w492 w495] -> w474
                        tunnel: [w491 w496] -> w473
                        tunnel: w470 -> [w490 _]
                        tunnel: w469 -> [w489 _]
                        tunnel: w467 -> [w488 _]
                        frame False {
                          n157 = call "Motors Move Relative.vi"("Axis Multiplier"=w488, "Axis"=w489, "error in"=w493, "VISA in"=w494, "Distance (mm)"=w490) -> ("error out"=w491:errorcluster, "VISA out"=w492:refnum<visa-resource-name>)  [unwired: 5 in]
                        }
                        frame True {
                        }
                      }
                      n158 = call "Motors Move Absolute.vi"("Axis Multiplier"=w468, "Axis"=w469, "error in"=w473, "VISA in"=w474, "Position (mm or degree)"=0.0) -> ("error out"=w471:errorcluster, "VISA out"=w472:refnum<visa-resource-name>)  [unwired: 5 in]
                    }
                    frame 3 {
                      w500 = u32 1 ("Axis Multiplier")
                      w502 = 4 ("Axis")
                      n159 = property on="Property Node" class="DigNum (strict)"(reference=w499) -> ("Value"=w501:u32)  [unwired: 1 in, 2 out]
                      n160 = call "Motors Status.vi"("error in"=w515, "VISA in"=w516, "Axis"=w502, "Axis Multiplier"=w501) -> ("error out"=w512:errorcluster, "VISA out"=w513:refnum<visa-resource-name>, "OS"=w520:i32, "Actual Position (mm or deg)"=w514:dbl)  [unwired: 3 in]
                      n161 = property on="Property Node" class="DigNum (strict)"(reference=w498, "Value"=w514) -> ()  [unwired: 1 in, 2 out]
                      n162 = call "Motors Position Redefine.vi"("Axis Multiplier"=w500, "Axis"=w502, "error in"=w512, "VISA in"=w513, "Position (mm or deg)"=w511) -> ("error out"=w506:errorcluster, "VISA out"=w507:refnum<visa-resource-name>)  [unwired: 5 in]
                      n163 = call "Motors Decipher Status.vi"("OS"=w520) -> ("Status"=w518:string)
                      n164 = property on="Property Node" class="Str"(reference=w497, "Value"=w518) -> ()  [unwired: 1 in, 2 out]
                      n165 = Equal?(x=w518, y="Idle") -> (x = y?=w517:bool)
                      n166 = case shown="False" w517 {
                        tunnel: w507 -> [w527 w529]
                        tunnel: w506 -> [w526 w528]
                        tunnel: [w525 w529] -> w505
                        tunnel: [w524 w528] -> w504
                        tunnel: "Steps to deactivate hard limit after finding datums" -> [w523 _]
                        tunnel: w502 -> [w522 _]
                        tunnel: w500 -> [w521 _]
                        frame False {
                          n167 = call "Motors Move Relative.vi"("Axis Multiplier"=w521, "Axis"=w522, "error in"=w526, "VISA in"=w527, "Distance (mm)"=w523) -> ("error out"=w524:errorcluster, "VISA out"=w525:refnum<visa-resource-name>)  [unwired: 5 in]
                        }
                        frame True {
                        }
                      }
                      n168 = call "Motors Move Absolute.vi"("Axis Multiplier"=w501, "Axis"=w502, "error in"=w504, "VISA in"=w505, "Position (mm or degree)"=0.0) -> ("error out"=w508:errorcluster, "VISA out"=w509:refnum<visa-resource-name>)  [unwired: 5 in]
                    }
                  }
                }
              }
              frame #2 {
                n169 = call <vilib>:"Unset Busy.vi"() -> ()  [unwired: 11 in, 1 out]
                n170 = property on="Property Node" class="Str"(reference=w531, "Value"="Running" ("Status")) -> (reference out=w530:refnum<vi>)  [unwired: 1 in, 1 out]
              }
            }
          }
        }
        n171 = case shown="True" w224 {
          tunnel: w262 -> [w1334 w1342]
          tunnel: w264 -> [w1333 w1345]
          tunnel: [w1334 w1343] -> w317
          tunnel: [w1333 w1344] -> w316
          tunnel: w179 -> [_ w1340]
          tunnel: w214 -> [_ w1337]
          tunnel: w213 -> [_ w1335]
          frame False {
          }
          frame True {
            n172 = property on="Property Node" class="DigNum (strict)"(reference=w1337) -> ("Value"=w1338:u32)  [unwired: 1 in, 2 out]
            n173 = property on="Property Node" class="DigNum (strict)"(reference=w1335) -> ("Value"=w1336:dbl)  [unwired: 1 in, 2 out]
            n174 = property on="Property Node" class="Bool (strict)"(reference=w1340, "Value"=FALSE) -> ()  [unwired: 1 in, 2 out]
            n175 = call "Motors Move Absolute.vi"("Axis Multiplier"=w1338, "Axis"=u32 1, "error in"=w1345, "VISA in"=w1342, "Position (mm or degree)"=w1336) -> ("error out"=w1344:errorcluster, "VISA out"=w1343:refnum<visa-resource-name>)  [unwired: 5 in]
          }
        }
        n176 = case shown="True" w210 {
          tunnel: w317 -> [w1321 w1329]
          tunnel: w316 -> [w1320 w1332]
          tunnel: [w1321 w1330] -> w315
          tunnel: [w1320 w1331] -> w314
          tunnel: w212 -> [_ w1325]
          tunnel: w211 -> [_ w1324]
          tunnel: w208 -> [_ w1322]
          frame False {
          }
          frame True {
            n177 = property on="Property Node" class="DigNum (strict)"(reference=w1325) -> ("Value"=w1327:u32)  [unwired: 1 in, 2 out]
            n178 = property on="Property Node" class="DigNum (strict)"(reference=w1324) -> ("Value"=w1326:dbl)  [unwired: 1 in, 2 out]
            n179 = property on="Property Node" class="Bool (strict)"(reference=w1322, "Value"=FALSE) -> ()  [unwired: 1 in, 2 out]
            n180 = call "Motors Move Absolute.vi"("Axis Multiplier"=w1327, "Axis"=u32 2, "error in"=w1332, "VISA in"=w1329, "Position (mm or degree)"=w1326) -> ("error out"=w1331:errorcluster, "VISA out"=w1330:refnum<visa-resource-name>)  [unwired: 5 in]
          }
        }
        n181 = case shown="True" w207 {
          tunnel: w315 -> [w1309 w1314]
          tunnel: w314 -> [w1308 w1319]
          tunnel: [w1309 w1317] -> w313
          tunnel: [w1308 w1318] -> w312
          tunnel: w205 -> [_ w1311]
          tunnel: w204 -> [_ w1310]
          frame False {
          }
          frame True {
            n182 = property on="Property Node" class="DigNum (strict)"() -> ("Value"=w1315:u32)  [unwired: 2 in, 2 out]
            n183 = property on="Property Node" class="DigNum (strict)"(reference=w1310) -> ("Value"=w1313:dbl)  [unwired: 1 in, 2 out]
            n184 = property on="Property Node" class="Bool (strict)"(reference=w1311, "Value"=FALSE) -> ()  [unwired: 1 in, 2 out]
            n185 = call "Motors Move Absolute.vi"("Axis Multiplier"=w1315, "Axis"=u32 3, "error in"=w1319, "VISA in"=w1314, "Position (mm or degree)"=w1313) -> ("error out"=w1318:errorcluster, "VISA out"=w1317:refnum<visa-resource-name>)  [unwired: 5 in]
          }
        }
        n186 = case shown="True" w203 {
          tunnel: w313 -> [w1295 w1304]
          tunnel: w312 -> [w1296 w1307]
          tunnel: [w1296 w1306] -> w310
          tunnel: [w1295 w1305] -> w311
          tunnel: w201 -> [_ w1299]
          tunnel: w198 -> [_ w1298]
          tunnel: w200 -> [_ w1297]
          frame False {
          }
          frame True {
            n187 = property on="Property Node" class="DigNum (strict)"(reference=w1297) -> ("Value"=w1301:dbl)  [unwired: 1 in, 2 out]
            n188 = property on="Property Node" class="DigNum (strict)"(reference=w1298) -> ("Value"=w1302:u32)  [unwired: 1 in, 2 out]
            n189 = property on="Property Node" class="Bool (strict)"(reference=w1299, "Value"=FALSE) -> ()  [unwired: 1 in, 2 out]
            n190 = call "Motors Move Absolute.vi"("Axis Multiplier"=w1302, "Axis"=u32 4, "error in"=w1307, "VISA in"=w1304, "Position (mm or degree)"=w1301) -> ("error out"=w1306:errorcluster, "VISA out"=w1305:refnum<visa-resource-name>)  [unwired: 5 in]
          }
        }
        n191 = case shown="True" w309 {
          tunnel: w311 -> [w1177 w1200]
          tunnel: w310 -> [w1176 w1199]
          tunnel: w197 -> [_ w1201]
          tunnel: [w1177 w1197] -> w308
          tunnel: [w1176 w1196] -> w307
          tunnel: w276 -> [_ w1198]
          tunnel: w195 -> [_ w1193]
          tunnel: w194 -> [_ w1192]
          tunnel: w193 -> [_ w1191]
          tunnel: w193 -> [_ w1190]
          tunnel: w192 -> [_ w1189]
          tunnel: w191 -> [_ w1188]
          tunnel: w190 -> [_ w1187]
          tunnel: w189 -> [_ w1186]
          tunnel: w188 -> [_ w1185]
          tunnel: w187 -> [_ w1184]
          tunnel: w186 -> [_ w1183]
          tunnel: w185 -> [_ w1182]
          tunnel: w178 -> [_ w1181]
          tunnel: w177 -> [_ w1180]
          tunnel: w176 -> [_ w1179]
          tunnel: w175 -> [_ w1178]
          frame False {
          }
          frame True {
            n192 = flat-sequence {
              tunnel: w1201 -> [w1218]
              tunnel: w1200 -> [w1217]
              tunnel: w1199 -> [w1216]
              tunnel: w1198 -> [w1215]
              tunnel: [w1214] -> w1195
              tunnel: [w1213] -> w1194
              tunnel: w1193 -> [w1212]
              tunnel: w1192 -> [w1211]
              tunnel: w1191 -> [w1210]
              tunnel: w1190 -> [w1209]
              tunnel: w1189 -> [w1208]
              tunnel: w1188 -> [w1207]
              tunnel: w1187 -> [w1206]
              tunnel: w1186 -> [w1205]
              tunnel: w1185 -> [w1204]
              tunnel: w1179 -> [w1203]
              tunnel: w1178 -> [w1202]
              tunnel: [w1293] -> w1196
              tunnel: [w1294] -> w1197
              tunnel: w1195 -> [w1294]
              tunnel: w1194 -> [w1293]
              tunnel: w1184 -> [_]
              tunnel: w1183 -> [_]
              tunnel: w1182 -> [_]
              tunnel: w1181 -> [w1290]
              tunnel: w1180 -> [w1289]
              frame #0 {
                n193 = case shown="True" w1218 {
                  tunnel: w1217 -> [w1228 w1260]
                  tunnel: w1216 -> [w1224 w1263]
                  tunnel: w1215 -> [w1227 w1268]
                  tunnel: [w1226 w1265] -> w1214
                  tunnel: [w1225 w1264] -> w1213
                  tunnel: w1212 -> [w1222 _]
                  tunnel: w1211 -> [w1220 _]
                  tunnel: w1210 -> [w1219 _]
                  tunnel: w1209 -> [_ w1256]
                  tunnel: w1208 -> [_ w1254]
                  tunnel: w1207 -> [_ w1253]
                  tunnel: w1206 -> [_ w1252]
                  tunnel: w1205 -> [_ w1251]
                  tunnel: w1204 -> [_ w1250]
                  tunnel: w1203 -> [_ w1249]
                  tunnel: w1202 -> [_ w1248]
                  frame False {
                    n194 = property on="Property Node" class="Bool (strict)"(reference=w1222) -> (reference out=w1221:refnum<vi>, "Value"=w1223:bool)  [unwired: 1 in, 1 out]
                    n195 = case shown="False" w1223 {
                      tunnel: w1228 -> [w1236 w1247]
                      tunnel: w1224 -> [w1241 w1246]
                      tunnel: w1227 -> [w1240 _]
                      tunnel: [w1238 w1247] -> w1226
                      tunnel: [w1239 w1246] -> w1225
                      tunnel: w1221 -> [w1232 _]
                      tunnel: w1220 -> [w1230 _]
                      tunnel: w1219 -> [w1229 _]
                      frame False {
                        n196 = property on="Property Node" class="DigNum (strict)"(reference=w1230) -> ("Value"=w1231:dbl)  [unwired: 1 in, 2 out]
                        n197 = property on="Property Node" class="Bool (strict)"(reference=w1232, "Value"=TRUE ("X Moving")) -> ()  [unwired: 1 in, 2 out]
                        n198 = case shown="True" w1240 {
                          tunnel: w1231 -> [w1242 w1244]
                          tunnel: [w1242 w1243] -> w1237
                          frame False {
                          }
                          frame True {
                            n199 = Multiply(x=w1244, y=-1.0) -> (x*y=w1243:dbl)
                          }
                        }
                        n200 = property on="Property Node" class="DigNum (strict)"(reference=w1229) -> ("Value"=w1234:u32)  [unwired: 1 in, 2 out]
                        n201 = call "Motors Move Relative.vi"("Axis Multiplier"=w1234, "Axis"=1, "error in"=w1241, "VISA in"=w1236, "Distance (mm)"=w1237) -> ("error out"=w1239:errorcluster, "VISA out"=w1238:refnum<visa-resource-name>)  [unwired: 5 in]
                      }
                      frame True {
                      }
                    }
                  }
                  frame True {
                    w1257 = 1 ("Axis")
                    n202 = property on="Property Node" class="DigNum (strict)"(reference=w1254) -> ("Value"=w1255:dbl)  [unwired: 1 in, 2 out]
                    n203 = property on="Property Node" class="DigNum (strict)"(reference=w1256) -> ("Value"=w1258:u32)  [unwired: 1 in, 2 out]
                    n204 = case shown="True" w1268 {
                      tunnel: w1255 -> [w1285 w1287]
                      tunnel: [w1285 w1286] -> w1261
                      frame False {
                      }
                      frame True {
                        n205 = Multiply(x=w1287, y=-1.0) -> (x*y=w1286:dbl)
                      }
                    }
                    n206 = call "Motors Move Constant Velocity.vi"("Axis Multiplier"=w1258, "Axis"=w1257, "error in"=w1263, "VISA in"=w1260, "Speed (mm/s)"=w1261) -> ("error out"=w1262:errorcluster, "VISA out"=w1259:refnum<visa-resource-name>)  [unwired: 5 in]
                    n207 = while {
                      tunnel: w1259 -> [w1274]
                      tunnel: [w1276] -> w1267
                      tunnel: w1262 -> [w1277]
                      tunnel: [w1275] -> w1266
                      tunnel: w1258 -> [w1273]
                      tunnel: w1253 -> [w1272]
                      tunnel: w1252 -> [_]
                      tunnel: w1251 -> [_]
                      tunnel: w1250 -> [w1271]
                      tunnel: w1249 -> [w1270]
                      tunnel: w1248 -> [w1269]
                      stop <- w1282 continue-if-true
                      n208 = property on="Property Node" class="Bool (strict)"(reference=w1270) -> ("Value"=w1283:bool)  [unwired: 1 in, 2 out]
                      n209 = property on="Property Node" class="Bool (strict)"(reference=w1269) -> ("Value"=w1284:bool)  [unwired: 1 in, 2 out]
                      n210 = Or(x=w1283, y=w1284) -> (x .or. y?=w1282:bool)
                      n211 = call "Motors Status.vi"("error in"=w1277, "VISA in"=w1274, "Axis"=1, "Axis Multiplier"=w1273) -> ("error out"=w1275:errorcluster, "VISA out"=w1276:refnum<visa-resource-name>, "OS"=w1280:i32, "Actual Position (mm or deg)"=w1278:dbl)  [unwired: 3 in]
                      n212 = call "Motors Decipher Status.vi"("OS"=w1280) -> ("Status"=w1279:string)
                      n213 = property on="Property Node" class="DigNum (strict)"(reference=w1272, "Value"=w1278) -> ()  [unwired: 1 in, 2 out]
                      n214 = property on="Property Node" class="Str"(reference=w1271, "Value"=w1279) -> ()  [unwired: 1 in, 2 out]
                    }
                    n215 = call "Motors Stop.vi"("error in"=w1266, "Axis"=w1257, "VISA in"=w1267) -> ("error out"=w1264:errorcluster, "VISA out"=w1265:refnum<visa-resource-name>)
                  }
                }
              }
              frame #1 {
                n216 = property on="Property Node" class="Bool (strict)"(reference=w1290, "Value"=FALSE) -> ()  [unwired: 1 in, 2 out]
                n217 = property on="Property Node" class="Bool (strict)"(reference=w1289, "Value"=FALSE) -> ()  [unwired: 1 in, 2 out]
              }
            }
          }
        }
        n218 = property on="Property Node" class="Bool (strict)"() -> ("Value"=w270:bool)  [unwired: 2 in, 2 out]
        n219 = property on="Property Node" class="Bool (strict)"() -> ("Value"=w271:bool)  [unwired: 2 in, 2 out]
        n220 = case shown="True" w306 {
          tunnel: w308 -> [w1106 w1113]
          tunnel: w307 -> [w1105 w1112]
          tunnel: w197 -> [_ w1114]
          tunnel: [w1106 w1111] -> w305
          tunnel: [w1105 w1110] -> w304
          tunnel: w274 -> [_ w1109]
          frame False {
          }
          frame True {
            n221 = flat-sequence {
              tunnel: w1114 -> [w1120]
              tunnel: w1113 -> [w1119]
              tunnel: w1112 -> [w1118]
              tunnel: w1109 -> [w1115]
              tunnel: [w1117] -> w1108
              tunnel: [w1116] -> w1107
              tunnel: [w1174] -> w1110
              tunnel: [w1175] -> w1111
              tunnel: w1108 -> [w1175]
              tunnel: w1107 -> [w1174]
              frame #0 {
                n222 = case shown="False" w1120 {
                  tunnel: w1119 -> [w1126 w1146]
                  tunnel: w1118 -> [w1125 w1149]
                  tunnel: [w1124 w1153] -> w1117
                  tunnel: [w1123 w1152] -> w1116
                  tunnel: w1115 -> [w1122 w1151]
                  frame False {
                    n223 = property on="Property Node" class="Bool (strict)"() -> ("Value"=w1121:bool)  [unwired: 2 in, 2 out]
                    n224 = case shown="False" w1121 {
                      tunnel: w1126 -> [w1131 w1142]
                      tunnel: w1125 -> [w1136 w1141]
                      tunnel: [w1132 w1142] -> w1124
                      tunnel: [w1135 w1141] -> w1123
                      tunnel: w1122 -> [w1134 _]
                      frame False {
                        n225 = property on="Property Node" class="Bool (strict)"("Value"=TRUE ("Y Moving")) -> ()  [unwired: 2 in, 2 out]
                        n226 = case shown="True" w1134 {
                          tunnel: "Delta Y (mm)" -> [w1137 w1139]
                          tunnel: [w1137 w1138] -> w1130
                          frame False {
                          }
                          frame True {
                            n227 = Multiply(x=w1139, y=-1.0) -> (x*y=w1138:dbl)
                          }
                        }
                        n228 = property on="Property Node" class="DigNum (strict)"() -> ("Value"=w1128:u32)  [unwired: 2 in, 2 out]
                        n229 = call "Motors Move Relative.vi"("Axis Multiplier"=w1128, "Axis"=2, "error in"=w1136, "VISA in"=w1131, "Distance (mm)"=w1130) -> ("error out"=w1135:errorcluster, "VISA out"=w1132:refnum<visa-resource-name>)  [unwired: 5 in]
                      }
                      frame True {
                      }
                    }
                  }
                  frame True {
                    w1143 = 2 ("Axis")
                    n230 = case shown="True" w1151 {
                      tunnel: "Y Speed (mm/s)" -> [w1168 w1170]
                      tunnel: [w1168 w1169] -> w1147
                      frame False {
                      }
                      frame True {
                        n231 = Multiply(x=w1170, y=-1.0) -> (x*y=w1169:dbl)
                      }
                    }
                    n232 = property on="Property Node" class="DigNum (strict)"() -> ("Value"=w1144:u32)  [unwired: 2 in, 2 out]
                    n233 = call "Motors Move Constant Velocity.vi"("Axis Multiplier"=w1144, "Axis"=w1143, "error in"=w1149, "VISA in"=w1146, "Speed (mm/s)"=w1147) -> ("error out"=w1148:errorcluster, "VISA out"=w1145:refnum<visa-resource-name>)  [unwired: 5 in]
                    n234 = while {
                      tunnel: w1145 -> [w1158]
                      tunnel: [w1157] -> w1155
                      tunnel: w1148 -> [w1160]
                      tunnel: [w1159] -> w1154
                      tunnel: w1144 -> [w1156]
                      stop <- w1167 continue-if-true
                      n235 = property on="Property Node" class="Bool (strict)"() -> ("Value"=w1166:bool)  [unwired: 2 in, 2 out]
                      n236 = property on="Property Node" class="Bool (strict)"() -> ("Value"=w1165:bool)  [unwired: 2 in, 2 out]
                      n237 = Or(x=w1166, y=w1165) -> (x .or. y?=w1167:bool)
                      n238 = call "Motors Status.vi"("error in"=w1160, "VISA in"=w1158, "Axis"=2, "Axis Multiplier"=w1156) -> ("error out"=w1159:errorcluster, "VISA out"=w1157:refnum<visa-resource-name>, "OS"=w1162:i32, "Actual Position (mm or deg)"=w1163:dbl)  [unwired: 3 in]
                      n239 = property on="Property Node" class="DigNum (strict)"("Value"=w1163) -> ()  [unwired: 2 in, 2 out]
                      n240 = call "Motors Decipher Status.vi"("OS"=w1162) -> ("Status"=w1161:string)
                      n241 = property on="Property Node" class="Str"("Value"=w1161) -> ()  [unwired: 2 in, 2 out]
                    }
                    n242 = call "Motors Stop.vi"("error in"=w1154, "Axis"=w1143, "VISA in"=w1155) -> ("error out"=w1152:errorcluster, "VISA out"=w1153:refnum<visa-resource-name>)
                  }
                }
              }
              frame #1 {
                n243 = property on="Property Node" class="Bool (strict)"("Value"=FALSE) -> ()  [unwired: 2 in, 2 out]
                n244 = property on="Property Node" class="Bool (strict)"("Value"=FALSE) -> ()  [unwired: 2 in, 2 out]
              }
            }
          }
        }
        n245 = case shown="True" w303 {
          tunnel: w305 -> [w992 w1011]
          tunnel: w304 -> [w991 w1004]
          tunnel: w197 -> [_ w1012]
          tunnel: [w992 w1010] -> w300
          tunnel: [w991 w1009] -> w301
          tunnel: w273 -> [_ w1008]
          tunnel: w182 -> [_ w1005]
          tunnel: w181 -> [_ w1003]
          tunnel: w180 -> [_ w1002]
          tunnel: w171 -> [_ w1001]
          tunnel: w174 -> [_ w1000]
          tunnel: w173 -> [_ w999]
          tunnel: w172 -> [_ w998]
          tunnel: w171 -> [_ w997]
          tunnel: w170 -> [_ w996]
          tunnel: w169 -> [_ w995]
          tunnel: w168 -> [_ w994]
          tunnel: w167 -> [_ w993]
          frame False {
          }
          frame True {
            n246 = flat-sequence {
              tunnel: w1012 -> [w1028]
              tunnel: w1011 -> [w1027]
              tunnel: w1008 -> [w1024]
              tunnel: [w1026] -> w1007
              tunnel: [w1025] -> w1006
              tunnel: w1005 -> [w1023]
              tunnel: w1004 -> [w1022]
              tunnel: w1003 -> [w1021]
              tunnel: w1002 -> [w1020]
              tunnel: w1001 -> [w1019]
              tunnel: w1000 -> [w1018]
              tunnel: w999 -> [w1017]
              tunnel: w998 -> [w1016]
              tunnel: w995 -> [w1015]
              tunnel: w994 -> [w1014]
              tunnel: w993 -> [w1013]
              tunnel: [w1103] -> w1009
              tunnel: [w1104] -> w1010
              tunnel: w1007 -> [w1104]
              tunnel: w1006 -> [w1103]
              tunnel: w997 -> [w1100]
              tunnel: w996 -> [w1099]
              frame #0 {
                n247 = case shown="False" w1028 {
                  tunnel: w1027 -> [w1038 w1070]
                  tunnel: w1022 -> [w1037 w1073]
                  tunnel: [w1036 w1076] -> w1026
                  tunnel: [w1035 w1075] -> w1025
                  tunnel: w1024 -> [w1034 w1064]
                  tunnel: w1023 -> [_ w1067]
                  tunnel: w1022 -> [_ w1066]
                  tunnel: w1021 -> [_ w1063]
                  tunnel: w1020 -> [_ w1062]
                  tunnel: w1019 -> [_ w1061]
                  tunnel: w1018 -> [_ w1060]
                  tunnel: w1017 -> [_ w1059]
                  tunnel: w1016 -> [_ w1058]
                  tunnel: w1015 -> [w1032 _]
                  tunnel: w1014 -> [w1031 _]
                  tunnel: w1013 -> [w1029 _]
                  frame False {
                    n248 = property on="Property Node" class="Bool (strict)"(reference=w1032) -> (reference out=w1030:refnum<vi>, "Value"=w1033:bool)  [unwired: 1 in, 1 out]
                    n249 = case shown="False" w1033 {
                      tunnel: w1038 -> [w1044 w1057]
                      tunnel: w1037 -> [w1051 w1056]
                      tunnel: [w1045 w1057] -> w1036
                      tunnel: [w1050 w1056] -> w1035
                      tunnel: w1034 -> [w1049 _]
                      tunnel: w1031 -> [w1041 _]
                      tunnel: w1030 -> [w1040 _]
                      tunnel: w1029 -> [w1039 _]
                      frame False {
                        n250 = property on="Property Node" class="DigNum (strict)"(reference=w1039) -> ("Value"=w1047:u32)  [unwired: 1 in, 2 out]
                        n251 = property on="Property Node" class="DigNum (strict)"(reference=w1041) -> ("Value"=w1042:dbl)  [unwired: 1 in, 2 out]
                        n252 = property on="Property Node" class="Bool (strict)"(reference=w1040, "Value"=TRUE ("Z Moving")) -> ()  [unwired: 1 in, 2 out]
                        n253 = case shown="True" w1049 {
                          tunnel: w1042 -> [w1052 w1054]
                          tunnel: [w1052 w1053] -> w1046
                          frame False {
                          }
                          frame True {
                            n254 = Multiply(x=w1054, y=-1.0) -> (x*y=w1053:dbl)
                          }
                        }
                        n255 = call "Motors Move Relative.vi"("Axis Multiplier"=w1047, "Axis"=3, "error in"=w1051, "VISA in"=w1044, "Distance (mm)"=w1046) -> ("error out"=w1050:errorcluster, "VISA out"=w1045:refnum<visa-resource-name>)  [unwired: 5 in]
                      }
                      frame True {
                      }
                    }
                  }
                  frame True {
                    w1072 = 3 ("Axis")
                    n256 = property on="Property Node" class="DigNum (strict)"(reference=w1067) -> ("Value"=w1068:u32)  [unwired: 1 in, 2 out]
                    n257 = property on="Property Node" class="DigNum (strict)"(reference=w1063, error in=w1066) -> ("Value"=w1065:dbl)  [unwired: 2 out]
                    n258 = case shown="True" w1064 {
                      tunnel: w1065 -> [w1095 w1097]
                      tunnel: [w1095 w1096] -> w1071
                      frame False {
                      }
                      frame True {
                        n259 = Multiply(x=w1097, y=-1.0) -> (x*y=w1096:dbl)
                      }
                    }
                    n260 = call "Motors Move Constant Velocity.vi"("Axis Multiplier"=w1068, "Axis"=w1072, "error in"=w1073, "VISA in"=w1070, "Speed (mm/s)"=w1071) -> ("error out"=w1074:errorcluster, "VISA out"=w1069:refnum<visa-resource-name>)  [unwired: 5 in]
                    n261 = while {
                      tunnel: w1069 -> [w1085]
                      tunnel: [w1084] -> w1078
                      tunnel: w1074 -> [w1087]
                      tunnel: [w1086] -> w1077
                      tunnel: w1068 -> [w1083]
                      tunnel: w1062 -> [w1082]
                      tunnel: w1061 -> [_]
                      tunnel: w1060 -> [w1081]
                      tunnel: w1059 -> [w1080]
                      tunnel: w1058 -> [w1079]
                      stop <- w1094 continue-if-true
                      n262 = property on="Property Node" class="Bool (strict)"(reference=w1081) -> ("Value"=w1093:bool)  [unwired: 1 in, 2 out]
                      n263 = property on="Property Node" class="Bool (strict)"(reference=w1080) -> ("Value"=w1092:bool)  [unwired: 1 in, 2 out]
                      n264 = Or(x=w1093, y=w1092) -> (x .or. y?=w1094:bool)
                      n265 = call "Motors Status.vi"("error in"=w1087, "VISA in"=w1085, "Axis"=3, "Axis Multiplier"=w1083) -> ("error out"=w1086:errorcluster, "VISA out"=w1084:refnum<visa-resource-name>, "OS"=w1089:i32, "Actual Position (mm or deg)"=w1090:dbl)  [unwired: 3 in]
                      n266 = property on="Property Node" class="DigNum (strict)"(reference=w1082, "Value"=w1090) -> ()  [unwired: 1 in, 2 out]
                      n267 = call "Motors Decipher Status.vi"("OS"=w1089) -> ("Status"=w1088:string)
                      n268 = property on="Property Node" class="Str"(reference=w1079, "Value"=w1088) -> ()  [unwired: 1 in, 2 out]
                    }
                    n269 = call "Motors Stop.vi"("error in"=w1077, "Axis"=w1072, "VISA in"=w1078) -> ("error out"=w1075:errorcluster, "VISA out"=w1076:refnum<visa-resource-name>)
                  }
                }
              }
              frame #1 {
                n270 = property on="Property Node" class="Bool (strict)"(reference=w1100, "Value"=FALSE) -> ()  [unwired: 1 in, 2 out]
                n271 = property on="Property Node" class="Bool (strict)"(reference=w1099, "Value"=FALSE) -> ()  [unwired: 1 in, 2 out]
              }
            }
          }
        }
        n272 = Or(x=w271, y=w270) -> (x .or. y?=w302:bool)
        n273 = case shown="True" w302 {
          tunnel: w300 -> [w921 w928]
          tunnel: w301 -> [w920 w927]
          tunnel: w197 -> [_ w929]
          tunnel: [w921 w926] -> w299
          tunnel: [w920 w925] -> w292
          tunnel: w270 -> [_ w924]
          frame False {
          }
          frame True {
            n274 = flat-sequence {
              tunnel: w929 -> [w935]
              tunnel: w928 -> [w934]
              tunnel: w927 -> [w933]
              tunnel: w924 -> [w930]
              tunnel: [w932] -> w923
              tunnel: [w931] -> w922
              tunnel: [w989] -> w925
              tunnel: [w990] -> w926
              tunnel: w923 -> [w990]
              tunnel: w922 -> [w989]
              frame #0 {
                n275 = case shown="True" w935 {
                  tunnel: w934 -> [w941 w962]
                  tunnel: w933 -> [w940 w963]
                  tunnel: [w939 w968] -> w932
                  tunnel: [w938 w967] -> w931
                  tunnel: w930 -> [w937 w966]
                  frame False {
                    n276 = property on="Property Node" class="Bool (strict)"() -> ("Value"=w936:bool)  [unwired: 2 in, 2 out]
                    n277 = case shown="False" w936 {
                      tunnel: w941 -> [w944 w957]
                      tunnel: w940 -> [w951 w956]
                      tunnel: [w945 w957] -> w939
                      tunnel: [w950 w956] -> w938
                      tunnel: w937 -> [w949 _]
                      frame False {
                        n278 = property on="Property Node" class="Bool (strict)"("Value"=TRUE ("Theta Moving")) -> ()  [unwired: 2 in, 2 out]
                        n279 = case shown="True" w949 {
                          tunnel: "Delta Theta (deg)" -> [w952 w954]
                          tunnel: [w952 w953] -> w943
                          frame False {
                          }
                          frame True {
                            n280 = Multiply(x=w954, y=-1.0) -> (x*y=w953:dbl)
                          }
                        }
                        n281 = property on="Property Node" class="DigNum (strict)"() -> ("Value"=w947:u32)  [unwired: 2 in, 2 out]
                        n282 = call "Motors Move Relative.vi"("Axis Multiplier"=w947, "Axis"=4, "error in"=w951, "VISA in"=w944, "Distance (mm)"=w943) -> ("error out"=w950:errorcluster, "VISA out"=w945:refnum<visa-resource-name>)  [unwired: 5 in]
                      }
                      frame True {
                      }
                    }
                  }
                  frame True {
                    w960 = 4 ("Axis")
                    n283 = case shown="True" w966 {
                      tunnel: "Theta Speed (deg/s)" -> [w983 w985]
                      tunnel: [w983 w984] -> w958
                      frame False {
                      }
                      frame True {
                        n284 = Multiply(x=w985, y=-1.0) -> (x*y=w984:dbl)
                      }
                    }
                    n285 = property on="Property Node" class="DigNum (strict)"() -> ("Value"=w959:u32)  [unwired: 2 in, 2 out]
                    n286 = call "Motors Move Constant Velocity.vi"("Axis Multiplier"=w959, "Axis"=w960, "error in"=w963, "VISA in"=w962, "Speed (mm/s)"=w958) -> ("error out"=w964:errorcluster, "VISA out"=w961:refnum<visa-resource-name>)  [unwired: 5 in]
                    n287 = while {
                      tunnel: w961 -> [w973]
                      tunnel: [w972] -> w970
                      tunnel: w964 -> [w975]
                      tunnel: [w974] -> w969
                      tunnel: w959 -> [w971]
                      stop <- w982 continue-if-true
                      n288 = property on="Property Node" class="Bool (strict)"() -> ("Value"=w981:bool)  [unwired: 2 in, 2 out]
                      n289 = property on="Property Node" class="Bool (strict)"() -> ("Value"=w980:bool)  [unwired: 2 in, 2 out]
                      n290 = Or(x=w981, y=w980) -> (x .or. y?=w982:bool)
                      n291 = call "Motors Status.vi"("error in"=w975, "VISA in"=w973, "Axis"=4, "Axis Multiplier"=w971) -> ("error out"=w974:errorcluster, "VISA out"=w972:refnum<visa-resource-name>, "OS"=w977:i32, "Actual Position (mm or deg)"=w978:dbl)  [unwired: 3 in]
                      n292 = property on="Property Node" class="DigNum (strict)"("Value"=w978) -> ()  [unwired: 2 in, 2 out]
                      n293 = call "Motors Decipher Status.vi"("OS"=w977) -> ("Status"=w976:string)
                      n294 = property on="Property Node" class="Str"("Value"=w976) -> ()  [unwired: 2 in, 2 out]
                    }
                    n295 = call "Motors Stop.vi"("error in"=w969, "Axis"=w960, "VISA in"=w970) -> ("error out"=w967:errorcluster, "VISA out"=w968:refnum<visa-resource-name>)
                  }
                }
              }
              frame #1 {
                n296 = property on="Property Node" class="Bool (strict)"("Value"=FALSE) -> ()  [unwired: 2 in, 2 out]
                n297 = property on="Property Node" class="Bool (strict)"("Value"=FALSE) -> ()  [unwired: 2 in, 2 out]
              }
            }
          }
        }
        n298 = case shown="True" "X Set Slew Speed" {
          tunnel: [w911 w914] -> w296
          tunnel: w299 -> [w911 w915]
          tunnel: [w910 w918] -> w293
          tunnel: w292 -> [w910 w919]
          frame False {
          }
          frame True {
            n299 = property on="Property Node" class="Bool (strict)"("Value"=TRUE ("Need to Update Motor Parameters")) -> ()  [unwired: 2 in, 2 out]
            n300 = property on="Property Node" class="DigNum (strict)"() -> ("Value"=w912:u32)  [unwired: 2 in, 2 out]
            n301 = call "Motors Move Speed.vi"("Speed (mm or degree/sec)"="(mm/s)", "error in"=w919, "VISA in"=w915, "Axis"=u32 1, "Axis Multiplier"=w912) -> ("error out"=w918:errorcluster, "VISA out"=w914:refnum<visa-resource-name>)  [unwired: 5 in]
          }
        }
        n302 = case shown="True" "Y Set Slew Speed" {
          tunnel: [w901 w905] -> w297
          tunnel: w296 -> [w901 w902]
          tunnel: [w900 w908] -> w294
          tunnel: w293 -> [w900 w909]
          frame False {
          }
          frame True {
            n303 = property on="Property Node" class="Bool (strict)"("Value"=TRUE ("Need to Update Motor Parameters")) -> ()  [unwired: 2 in, 2 out]
            n304 = property on="Property Node" class="DigNum (strict)"() -> ("Value"=w903:u32)  [unwired: 2 in, 2 out]
            n305 = call "Motors Move Speed.vi"("Speed (mm or degree/sec)"="(mm/s) 3", "error in"=w909, "VISA in"=w902, "Axis"=u32 2, "Axis Multiplier"=w903) -> ("error out"=w908:errorcluster, "VISA out"=w905:refnum<visa-resource-name>)  [unwired: 5 in]
          }
        }
        n306 = case shown="True" "Z Set Slew Speed" {
          tunnel: [w891 w895] -> w298
          tunnel: w297 -> [w891 w894]
          tunnel: [w890 w898] -> w295
          tunnel: w294 -> [w890 w899]
          frame False {
          }
          frame True {
            n307 = property on="Property Node" class="Bool (strict)"("Value"=TRUE ("Need to Update Motor Parameters")) -> ()  [unwired: 2 in, 2 out]
            n308 = property on="Property Node" class="DigNum (strict)"() -> ("Value"=w892:u32)  [unwired: 2 in, 2 out]
            n309 = call "Motors Move Speed.vi"("Speed (mm or degree/sec)"="(mm/s) 2", "error in"=w899, "VISA in"=w894, "Axis"=u32 3, "Axis Multiplier"=w892) -> ("error out"=w898:errorcluster, "VISA out"=w895:refnum<visa-resource-name>)  [unwired: 5 in]
          }
        }
        n310 = case shown="True" "Theta Set Slew Speed" {
          tunnel: [w881 w885] -> w286
          tunnel: w298 -> [w881 w884]
          tunnel: [w880 w886] -> w287
          tunnel: w295 -> [w880 w889]
          frame False {
          }
          frame True {
            n311 = property on="Property Node" class="Bool (strict)"("Value"=TRUE ("Need to Update Motor Parameters")) -> ()  [unwired: 2 in, 2 out]
            n312 = property on="Property Node" class="DigNum (strict)"() -> ("Value"=w882:u32)  [unwired: 2 in, 2 out]
            n313 = call "Motors Move Speed.vi"("Speed (mm or degree/sec)"="(degrees/s)", "error in"=w889, "VISA in"=w884, "Axis"=u32 4, "Axis Multiplier"=w882) -> ("error out"=w886:errorcluster, "VISA out"=w885:refnum<visa-resource-name>)  [unwired: 5 in]
          }
        }
        n314 = Quotient & Remainder(x=w260, y=4) -> (x-y*floor(x/y)=w284:i32)  [unwired: 1 out]
        n315 = case shown="2" w284 {
          tunnel: w287 -> [w764 w778 w791 w806]
          tunnel: w286 -> [w765 w779 w793 w807]
          tunnel: [w763 w776 w790 w805] -> w281
          tunnel: [w762 w777 w792 w804] -> w280
          frame 0, Default {
            n316 = property on="Property Node" class="DigNum (strict)"() -> ("Value"=w761:u32)  [unwired: 2 in, 2 out]
            n317 = call "Motors Status.vi"("error in"=w764, "VISA in"=w765, "Axis"=1, "Axis Multiplier"=w761) -> ("error out"=w763:errorcluster, "VISA out"=w762:refnum<visa-resource-name>, "OS"=w771:i32, "Actual Position (mm or deg)"=w766:dbl)  [unwired: 3 in]
            n318 = property on="Property Node" class="DigNum (strict)"("Value"=w766) -> ()  [unwired: 2 in, 2 out]
            n319 = call "Motors Decipher Status.vi"("OS"=w771) -> ("Status"=w770:string)
            n320 = property on="Property Node" class="Str"("Value"=w770) -> ()  [unwired: 2 in, 2 out]
            n321 = Equal?(x=w770, y="Idle") -> (x = y?=w768:bool)
            n322 = case shown="False" w768 {
              tunnel: [TRUE FALSE] -> w767
              frame False {
              }
              frame True {
              }
            }
            n323 = property on="Property Node" class="Bool (strict)"("Value"=w767) -> ()  [unwired: 2 in, 2 out]
          }
          frame 1 {
            n324 = property on="Property Node" class="DigNum (strict)"() -> ("Value"=w775:u32)  [unwired: 2 in, 2 out]
            n325 = call "Motors Status.vi"("error in"=w778, "VISA in"=w779, "Axis"=2, "Axis Multiplier"=w775) -> ("error out"=w776:errorcluster, "VISA out"=w777:refnum<visa-resource-name>, "OS"=w784:i32, "Actual Position (mm or deg)"=w785:dbl)  [unwired: 3 in]
            n326 = property on="Property Node" class="DigNum (strict)"("Value"=w785) -> ()  [unwired: 2 in, 2 out]
            n327 = call "Motors Decipher Status.vi"("OS"=w784) -> ("Status"=w782:string)
            n328 = property on="Property Node" class="Str"("Value"=w782) -> ()  [unwired: 2 in, 2 out]
            n329 = Equal?(x=w782, y="Idle") -> (x = y?=w781:bool)
            n330 = case shown="False" w781 {
              tunnel: [TRUE FALSE] -> w780
              frame False {
              }
              frame True {
              }
            }
            n331 = property on="Property Node" class="Bool (strict)"("Value"=w780) -> ()  [unwired: 2 in, 2 out]
          }
          frame 2 {
            n332 = property on="Property Node" class="DigNum (strict)"() -> ("Value"=w789:u32)  [unwired: 2 in, 2 out]
            n333 = call "Motors Status.vi"("error in"=w791, "VISA in"=w793, "Axis"=3, "Axis Multiplier"=w789) -> ("error out"=w790:errorcluster, "VISA out"=w792:refnum<visa-resource-name>, "OS"=w798:i32, "Actual Position (mm or deg)"=w799:dbl)  [unwired: 3 in]
            n334 = property on="Property Node" class="DigNum (strict)"("Value"=w799) -> ()  [unwired: 2 in, 2 out]
            n335 = call "Motors Decipher Status.vi"("OS"=w798) -> ("Status"=w796:string)
            n336 = property on="Property Node" class="Str"("Value"=w796) -> ()  [unwired: 2 in, 2 out]
            n337 = Equal?(x=w796, y="Idle") -> (x = y?=w795:bool)
            n338 = case shown="False" w795 {
              tunnel: [TRUE FALSE] -> w794
              frame False {
              }
              frame True {
              }
            }
            n339 = property on="Property Node" class="Bool (strict)"("Value"=w794) -> ()  [unwired: 2 in, 2 out]
          }
          frame 3 {
            n340 = property on="Property Node" class="DigNum (strict)"() -> ("Value"=w803:u32)  [unwired: 2 in, 2 out]
            n341 = call "Motors Status.vi"("error in"=w806, "VISA in"=w807, "Axis"=4, "Axis Multiplier"=w803) -> ("error out"=w805:errorcluster, "VISA out"=w804:refnum<visa-resource-name>, "OS"=w812:i32, "Actual Position (mm or deg)"=w813:dbl)  [unwired: 3 in]
            n342 = property on="Property Node" class="DigNum (strict)"("Value"=w813) -> ()  [unwired: 2 in, 2 out]
            n343 = call "Motors Decipher Status.vi"("OS"=w812) -> ("Status"=w810:string)
            n344 = property on="Property Node" class="Str"("Value"=w810) -> ()  [unwired: 2 in, 2 out]
            n345 = Equal?(x=w810, y="Idle") -> (x = y?=w809:bool)
            n346 = case shown="True" w809 {
              tunnel: [TRUE FALSE] -> w808
              frame False {
              }
              frame True {
              }
            }
            n347 = property on="Property Node" class="Bool (strict)"("Value"=w808) -> ()  [unwired: 2 in, 2 out]
          }
        }
        n348 = case shown="True" "Go To Saved Position" {
          tunnel: w281 -> [w730 w732]
          tunnel: w280 -> [w729 w738]
          tunnel: [w730 w751] -> w279
          tunnel: [w729 w750] -> w278
          frame False {
          }
          frame True {
            w748 = 4 ("index (row)")
            w746 = 3 ("index (row)")
            w743 = 2 ("index (row)")
            w740 = 1 ("index (row)")
            n349 = property on="Property Node" class="Path"() -> ("Value"=w733:path)  [unwired: 2 in, 2 out]
            n350 = call "Motors Position Load.vi"("error in"=w732, "file path"=w733) -> ("error out"=w731:errorcluster, "Positions"=w755:string[][])
            n351 = property on="Property Node" class="DigNum (strict)"() -> ("Value"=w737:u32)  [unwired: 2 in, 2 out]
            n352 = Index Array(array=w755, index (row)=w748, index (col)="Defined Positions") -> (element=w756:string)
            n353 = Index Array(array=w755, index (row)=w746, index (col)="Defined Positions") -> (element=w757:string)
            n354 = Index Array(array=w755, index (row)=w743, index (col)="Defined Positions") -> (element=w759:string)
            n355 = Index Array(array=w755, index (row)=w740, index (col)="Defined Positions") -> (element=w760:string)
            n356 = Fract/Exp String To Number(string=w756) -> (number=w749:dbl)  [unwired: 3 in, 1 out]
            n357 = Fract/Exp String To Number(string=w757) -> (number=w745:dbl)  [unwired: 3 in, 1 out]
            n358 = Fract/Exp String To Number(string=w759) -> (number=w742:dbl)  [unwired: 3 in, 1 out]
            n359 = Fract/Exp String To Number(string=w760) -> (number=w739:dbl)  [unwired: 3 in, 1 out]
            n360 = property on="Property Node" class="DigNum (strict)"() -> ("Value"=w736:u32)  [unwired: 2 in, 2 out]
            n361 = property on="Property Node" class="DigNum (strict)"() -> ("Value"=w735:u32)  [unwired: 2 in, 2 out]
            n362 = call "Motors Move Absolute.vi"("Axis Multiplier"=w737, "Axis"=w740, "error in"=w731, "VISA in"=w738, "Position (mm or degree)"=w739) -> ("error out"=w758:errorcluster, "VISA out"=w741:refnum<visa-resource-name>)  [unwired: 5 in]
            n363 = property on="Property Node" class="DigNum (strict)"() -> ("Value"=w734:u32)  [unwired: 2 in, 2 out]
            n364 = call "Motors Move Absolute.vi"("Axis Multiplier"=w736, "Axis"=w743, "error in"=w758, "VISA in"=w741, "Position (mm or degree)"=w742) -> ("error out"=w754:errorcluster, "VISA out"=w744:refnum<visa-resource-name>)  [unwired: 5 in]
            n365 = call "Motors Move Absolute.vi"("Axis Multiplier"=w735, "Axis"=w746, "error in"=w754, "VISA in"=w744, "Position (mm or degree)"=w745) -> ("error out"=w753:errorcluster, "VISA out"=w747:refnum<visa-resource-name>)  [unwired: 5 in]
            n366 = call "Motors Move Absolute.vi"("Axis Multiplier"=w734, "Axis"=w748, "error in"=w753, "VISA in"=w747, "Position (mm or degree)"=w749) -> ("error out"=w751:errorcluster, "VISA out"=w750:refnum<visa-resource-name>)  [unwired: 5 in]
          }
        }
        n367 = property on="Property Node" class="Bool (strict)"() -> ("Value"=w285:bool)  [unwired: 2 in, 2 out]
        n368 = case shown="True" w285 {
          tunnel: w279 -> [w818 w821]
          tunnel: w278 -> [w817 w822]
          tunnel: [w817 w820] -> _
          tunnel: [w818 w819] -> w267
          frame False {
          }
          frame True {
            n369 = property on="Property Node" class="Bool (strict)"("Value"=FALSE ("Need to Update Motor Parameters")) -> ()  [unwired: 2 in, 2 out]
            n370 = flat-sequence {
              tunnel: w822 -> [w828]
              tunnel: w821 -> [w827]
              tunnel: [w826] -> w820
              tunnel: [w825] -> w819
              frame #0 {
                n371 = call <vilib>:"Set Busy.vi"() -> ()  [unwired: 10 in, 2 out]
                n372 = property on="Property Node" class="Str"("Value"="Updating Motor Parameters\nThis Should Take About 5 Seconds" ("Status Theta")) -> ()  [unwired: 2 in, 2 out]
              }
              frame #1 {
                n373 = call "Motors Status Verbose.vi"("Axis"=1, "VISA in"=w828, "error in"=w827) -> ("Slew Speed (mm or deg/s)"=w847:dbl, "Jogger Normal Speed (mm or deg/s)"=w848:dbl, "Jogger Fast Speed (mm or deg/s)"=w849:dbl, "Actual Position (mm or deg)"=w864:dbl, "OS"=w835:i32, "Mode"=w873:string, "VISA out"=w853:refnum<visa-resource-name>, "Creep Speed (mm or deg/s)"=w878:dbl, "error out"=w832:errorcluster)  [unwired: 4 in]
                n374 = property on="Property Node" class="Str"("Value"=w873) -> ()  [unwired: 2 in, 2 out]
                n375 = property on="Property Node" class="DigNum (strict)"("Value"=w847) -> ()  [unwired: 2 in, 2 out]
                n376 = property on="Property Node" class="DigNum (strict)"("Value"=w848) -> ()  [unwired: 2 in, 2 out]
                n377 = property on="Property Node" class="DigNum (strict)"("Value"=w849) -> ()  [unwired: 2 in, 2 out]
                n378 = property on="Property Node" class="DigNum (strict)"("Value"=w864) -> ()  [unwired: 2 in, 2 out]
                n379 = call "Motors Decipher Status.vi"("OS"=w835) -> ("Status"=w875:string)
                n380 = call "Motors Status Verbose.vi"("Axis"=2, "VISA in"=w853, "error in"=w832) -> ("Slew Speed (mm or deg/s)"=w850:dbl, "Jogger Normal Speed (mm or deg/s)"=w851:dbl, "Jogger Fast Speed (mm or deg/s)"=w852:dbl, "Actual Position (mm or deg)"=w865:dbl, "OS"=w836:i32, "Mode"=w874:string, "VISA out"=w854:refnum<visa-resource-name>, "Creep Speed (mm or deg/s)"=w843:dbl, "error out"=w833:errorcluster)  [unwired: 4 in]
                n381 = property on="(mm/s)" class="DigNum (strict)"("Minimum"=w878) -> ()  [unwired: 2 in, 2 out]
                n382 = property on="Property Node" class="Str"("Value"=w875) -> ()  [unwired: 2 in, 2 out]
                n383 = property on="Property Node" class="Str"("Value"=w874) -> ()  [unwired: 2 in, 2 out]
                n384 = property on="Property Node" class="DigNum (strict)"("Value"=w850) -> ()  [unwired: 2 in, 2 out]
                n385 = property on="Property Node" class="DigNum (strict)"("Value"=w851) -> ()  [unwired: 2 in, 2 out]
                n386 = property on="Property Node" class="DigNum (strict)"("Value"=w852) -> ()  [unwired: 2 in, 2 out]
                n387 = property on="Property Node" class="DigNum (strict)"("Value"=w865) -> ()  [unwired: 2 in, 2 out]
                n388 = call "Motors Decipher Status.vi"("OS"=w836) -> ("Status"=w866:string)
                n389 = call "Motors Status Verbose.vi"("Axis"=3, "VISA in"=w854, "error in"=w833) -> ("Slew Speed (mm or deg/s)"=w863:dbl, "Jogger Normal Speed (mm or deg/s)"=w862:dbl, "Jogger Fast Speed (mm or deg/s)"=w861:dbl, "Actual Position (mm or deg)"=w860:dbl, "OS"=w837:i32, "Mode"=w867:string, "VISA out"=w855:refnum<visa-resource-name>, "Creep Speed (mm or deg/s)"=w844:dbl, "error out"=w834:errorcluster)  [unwired: 4 in]
                n390 = property on="(mm/s) 3" class="DigNum (strict)"("Minimum"=w843) -> ()  [unwired: 2 in, 2 out]
                n391 = Not Equal?(x=w875, y="Idle") -> (x != y?=w856:bool)
                n392 = property on="Property Node" class="Str"("Value"=w866) -> ()  [unwired: 2 in, 2 out]
                n393 = property on="Property Node" class="Str"("Value"=w867) -> ()  [unwired: 2 in, 2 out]
                n394 = property on="Property Node" class="DigNum (strict)"("Value"=w863) -> ()  [unwired: 2 in, 2 out]
                n395 = property on="Property Node" class="DigNum (strict)"("Value"=w862) -> ()  [unwired: 2 in, 2 out]
                n396 = property on="Property Node" class="DigNum (strict)"("Value"=w861) -> ()  [unwired: 2 in, 2 out]
                n397 = property on="Property Node" class="DigNum (strict)"("Value"=w860) -> ()  [unwired: 2 in, 2 out]
                n398 = property on="Property Node" class="Bool (strict)"("Value"=w856) -> ()  [unwired: 2 in, 2 out]
                n399 = property on="(mm/s) 2" class="DigNum (strict)"("Minimum"=w844) -> ()  [unwired: 2 in, 2 out]
                n400 = call "Motors Status Verbose.vi"("Axis"=4, "VISA in"=w855, "error in"=w834) -> ("Slew Speed (mm or deg/s)"=w869:dbl, "Jogger Normal Speed (mm or deg/s)"=w870:dbl, "Jogger Fast Speed (mm or deg/s)"=w871:dbl, "Actual Position (mm or deg)"=w872:dbl, "OS"=w838:i32, "Mode"=w876:string, "VISA out"=w826:refnum<visa-resource-name>, "Creep Speed (mm or deg/s)"=w845:dbl, "error out"=w825:errorcluster)  [unwired: 4 in]
                n401 = call "Motors Decipher Status.vi"("OS"=w837) -> ("Status"=w868:string)
                n402 = Not Equal?(x=w866, y="Idle") -> (x != y?=w857:bool)
                n403 = property on="Property Node" class="DigNum (strict)"("Value"=w869) -> ()  [unwired: 2 in, 2 out]
                n404 = property on="Property Node" class="DigNum (strict)"("Value"=w870) -> ()  [unwired: 2 in, 2 out]
                n405 = property on="Property Node" class="DigNum (strict)"("Value"=w871) -> ()  [unwired: 2 in, 2 out]
                n406 = property on="Property Node" class="DigNum (strict)"("Value"=w872) -> ()  [unwired: 2 in, 2 out]
                n407 = property on="Property Node" class="Str"("Value"=w868) -> ()  [unwired: 2 in, 2 out]
                n408 = property on="Property Node" class="Str"("Value"=w876) -> ()  [unwired: 2 in, 2 out]
                n409 = property on="(degrees/s)" class="DigNum (strict)"("Minimum"=w845) -> ()  [unwired: 2 in, 2 out]
                n410 = call "Motors Decipher Status.vi"("OS"=w838) -> ("Status"=w877:string)
                n411 = property on="Property Node" class="Bool (strict)"("Value"=w857) -> ()  [unwired: 2 in, 2 out]
                n412 = property on="Property Node" class="Str"("Value"=w877) -> ()  [unwired: 2 in, 2 out]
                n413 = Not Equal?(x=w868, y="Idle") -> (x != y?=w858:bool)
                n414 = Not Equal?(x=w877, y="Idle") -> (x != y?=w859:bool)
                n415 = property on="Property Node" class="Bool (strict)"("Value"=w858) -> ()  [unwired: 2 in, 2 out]
                n416 = property on="Property Node" class="Bool (strict)"("Value"=w859) -> ()  [unwired: 2 in, 2 out]
              }
              frame #2 {
                n417 = call <vilib>:"Unset Busy.vi"() -> ()  [unwired: 11 in, 1 out]
                n418 = property on="Property Node" class="Str"("Value"="Running" ("Status Theta")) -> ()  [unwired: 2 in, 2 out]
              }
            }
          }
        }
        n419 = property on="Property Node" class="Clust (strict)"("Value"=w267) -> ()  [unwired: 2 in, 2 out]
        "Loop i" <- w260
      }
    }
  }
  n420 = property on="Property Node" class="Bool (strict)"(reference=w69, "Value"=w75) -> ()  [unwired: 1 in, 2 out]
